vi "lv_icon.vi"(10 "Color icon in":T2, 11 "BW icon in":T2) -> (0 "Error code out":i32=43, 2 "Color icon out":T2, 3 "BW icon out":T2)   [LabVIEW 2020, in "lv_icon.lvlib"]
doc: "<p>Display this dialog box in one of the following ways:</p>\n\n<ul>\n<li>Double-click the <a href=\"nihelplauncher://docs/csh?context=lvcore_lvconcepts_using_icons\">icon</a> in the upper right corner of the front panel window, block diagram window, or <a href=\"nihelplauncher://docs/csh?context=lvcore_lvconcepts_custom_cont_ind_type\">Control Editor</a> window.</li>\n<li>Right-click the icon in the upper right corner of the front panel window, block diagram window, or <strong>Control Editor</strong> window and select <strong>Edit Icon</strong> from the shortcut menu.</li>\n<li>Select <strong>File<span class=\"U+187\">>></span>VI Properties</strong> or <strong>File<span class=\"U+187\">>></span>Control Properties</strong> to display the <a href=\"nihelplauncher://docs/csh?context=lvcore_lvdialog_vi_properties_dialog_box\">VI Properties</a> dialog box or <strong>Control Properties</strong> dialog box, respectively. Then select <strong>General</strong> from the <strong>Category</strong> pull-down menu and click the <strong>Edit Icon</strong> button.</li>\n<li>Right-click a project library, statechart, class, or XControl item in the <a href=\"nihelplauncher://docs/csh?context=lvcore_lvconcepts_using_labview_projects\">Project Explorer</a> window and select <strong> Properties</strong> from the shortcut menu to display the corresponding <strong>Properties</strong> dialog box. Then click the <strong>Edit</strong> button on the <strong>General Settings</strong> page.</li>\n</ul>\n\n<p>Use this dialog box to <a href=\"nihelplauncher://docs/csh?context=lvcore_lvhowto_creating_icons\">create and edit icons</a>.</p>"
uses:
  lv_icon.lvlib
  NIIconEditor/Class/Ants/Ants.lvclass
  NIIconEditor/Class/FakedArray/FakedArray.lvclass
  vi.lib/LabVIEW Icon API/lv_icon/Classes/Icon/Icon.lvclass
  NIIconEditor/Class/Icon Library/Glyph.lvclass
  NIIconEditor/Class/Settings/Settings.lvclass
  NIIconEditor/Class/Tools/Tools Paint.lvclass
  vi.lib/LabVIEW Icon API/lv_icon/Controls/Pathes.ctl
  NIIconEditor/History/History.lvlib
  <vilib>/Utility/miscctls.llb/LVPoint32TypeDef.ctl
  NIIconEditor/Controls/Tools.ctl
  NIIconEditor/Controls/References Cluster.ctl
  NIIconEditor/Controls/Path&Icon.ctl
  vi.lib/LabVIEW Icon API/lv_icon/Controls/Graphic.ctl
  NIIconEditor/Global Variables/Data.vi
  <vilib>/Utility/miscctls.llb/LVMenuShortCut.ctl
  <resource>/plugins/IconEditor/Icon Editor Invoker Type.ctl
  NIIconEditor/Controls/Circle.ctl
  NIIconEditor/Controls/Dropper.ctl
  NIIconEditor/Controls/FCircle.ctl
  NIIconEditor/Controls/Fill.ctl
  NIIconEditor/Controls/FRect.ctl
  NIIconEditor/Controls/Line.ctl
  NIIconEditor/Controls/Move.ctl
  NIIconEditor/Controls/Pen.ctl
  NIIconEditor/Controls/Rubber.ctl
  NIIconEditor/Controls/Selection.ctl
  NIIconEditor/Controls/Text.ctl
  NIIconEditor/Controls/Rotate.ctl
  NIIconEditor/Controls/Flip.ctl
  vi.lib/LabVIEW Icon API/lv_icon/Controls/IEColor.ctl
  NIIconEditor/Controls/ColorChange.ctl
  NIIconEditor/Controls/Framework Templates.ctl
  NIIconEditor/Controls/TextMarker.ctl
  <vilib>/picture/picture.llb/imagedata.ctl
  vi.lib/LabVIEW Icon API/lv_icon/Controls/BodyText.ctl
  vi.lib/LabVIEW Icon API/lv_icon/Controls/Layer.ctl
  vi.lib/LabVIEW Icon API/lv_icon/Controls/Font.ctl
  NIIconEditor/Controls/LayerList.ctl
  vi.lib/LabVIEW Icon API/lv_icon/Controls/Alignment.ctl
  NIIconEditor/Controls/Arrow Up.ctl
  NIIconEditor/Controls/Arrow Down.ctl
  NIIconEditor/Controls/DeleteLayer.ctl
  NIIconEditor/Controls/NewLayer.ctl
  NIIconEditor/Controls/IERect.ctl
  NIIconEditor/Controls/Refresh.ctl
panel:
  out "LabVIEW Icon out":string
  in  "LabVIEW Icon in":string
  out "Terminals":picture
  out "Preview2":picture
  out "TextMarker":T1="^"
  in  "Help":bool
  in  "Cancel":bool
  in  "OK":bool
  out "XYZ":string="X: 14\nY: 31\nZ: 1"
  out "RGB":string="R: 0\nG: 0\nB: 0"
  out "Icon":picture
  out "Clipboard":picture
  in  "Tab Control":T3(tab)
  in  "refreshTemplates":T4
  out "templates path str":string
  in  "Templates":string(tree)="<All>"
  in  "Filter templates by keyword":string
  in  "Framework Templates":T5={"Scrollbar"=0, "Path & Icon 1"={"Rectangle"={"left"=0, "top"=0, "right"=32, "bottom"=32}, "Path"=path "C:/Users/tsandris/Documents/LabVIEW Data/Icon Templates/VI/Frameworks/_blank.png", "Image"=bytes[0], "Filter"="VI\\Frameworks", "FileName"="_blank"}, "Path & Icon 2"={"Rectangle"={"left"=0, "top"=0, "right"=32, "bottom"=32}, "Path"=path "C:/Users/tsandris/Documents/LabVIEW Data/Icon Templates/Library/Frameworks/_blank.png", "Image"=bytes[0], "Filter"="Library\\Frameworks", "FileName"="_blank"}, "Path & Icon 3"={"Rectangle"={"left"=0, "top"=0, "right"=0, "bottom"=0}, "Path"=path "", "Image"=bytes[0], "Filter"="", "FileName"=""}, "Path & Icon 4"={"Rectangle"={"left"=0, "top"=0, "right"=0, "bottom"=0}, "Path"=path "", "Image"=bytes[0], "Filter"="", "FileName"=""}, "Path & Icon 5"={"Rectangle"={"left"=0, "top"=0, "right"=0, "bottom"=0}, "Path"=path "", "Image"=bytes[0], "Filter"="", "FileName"=""}, "Path & Icon 6"={"Rectangle"={"left"=0, "top"=0, "right"=0, "bottom"=0}, "Path"=path "", "Image"=bytes[0], "Filter"="", "FileName"=""}, "Path & Icon 7"={"Rectangle"={"left"=0, "top"=0, "right"=0, "bottom"=0}, "Path"=path "", "Image"=bytes[0], "Filter"="", "FileName"=""}, "Path & Icon 8"={"Rectangle"={"left"=0, "top"=0, "right"=0, "bottom"=0}, "Path"=path "", "Image"=bytes[0], "Filter"="", "FileName"=""}, "Path & Icon 9"={"Rectangle"={"left"=0, "top"=0, "right"=0, "bottom"=0}, "Path"=path "", "Image"=bytes[0], "Filter"="", "FileName"=""}, "Path & Icon 10"={"Rectangle"={"left"=0, "top"=0, "right"=0, "bottom"=0}, "Path"=path "", "Image"=bytes[0], "Filter"="", "FileName"=""}, "Path & Icon 11"={"Rectangle"={"left"=0, "top"=0, "right"=0, "bottom"=0}, "Path"=path "", "Image"=bytes[0], "Filter"="", "FileName"=""}, "Path & Icon 12"={"Rectangle"={"left"=0, "top"=0, "right"=0, "bottom"=0}, "Path"=path "", "Image"=bytes[0], "Filter"="", "FileName"=""}, "Path & Icon 13"={"Rectangle"={"left"=0, "top"=0, "right"=0, "bottom"=0}, "Path"=path "", "Image"=bytes[0], "Filter"="", "FileName"=""}, "Path & Icon 14"={"Rectangle"={"left"=0, "top"=0, "right"=0, "bottom"=0}, "Path"=path "", "Image"=bytes[0], "Filter"="", "FileName"=""}, "Path & Icon 15"={"Rectangle"={"left"=0, "top"=0, "right"=0, "bottom"=0}, "Path"=path "", "Image"=bytes[0], "Filter"="", "FileName"=""}, "Path & Icon 16"={"Rectangle"={"left"=0, "top"=0, "right"=0, "bottom"=0}, "Path"=path "", "Image"=bytes[0], "Filter"="", "FileName"=""}, "Path & Icon 17"={"Rectangle"={"left"=0, "top"=0, "right"=0, "bottom"=0}, "Path"=path "", "Image"=bytes[0], "Filter"="", "FileName"=""}, "Path & Icon 18"={"Rectangle"={"left"=0, "top"=0, "right"=0, "bottom"=0}, "Path"=path "", "Image"=bytes[0], "Filter"="", "FileName"=""}, "Path & Icon 19"={"Rectangle"={"left"=0, "top"=0, "right"=0, "bottom"=0}, "Path"=path "", "Image"=bytes[0], "Filter"="", "FileName"=""}, "Path & Icon 20"={"Rectangle"={"left"=0, "top"=0, "right"=0, "bottom"=0}, "Path"=path "", "Image"=bytes[0], "Filter"="", "FileName"=""}, "Path & Icon 21"={"Rectangle"={"left"=0, "top"=0, "right"=0, "bottom"=0}, "Path"=path "", "Image"=bytes[0], "Filter"="", "FileName"=""}, "Path & Icon 22"={"Rectangle"={"left"=0, "top"=0, "right"=0, "bottom"=0}, "Path"=path "", "Image"=bytes[0], "Filter"="", "FileName"=""}, "Path & Icon 23"={"Rectangle"={"left"=0, "top"=0, "right"=0, "bottom"=0}, "Path"=path "", "Image"=bytes[0], "Filter"="", "FileName"=""}, "Path & Icon 24"={"Rectangle"={"left"=0, "top"=0, "right"=0, "bottom"=0}, "Path"=path "", "Image"=bytes[0], "Filter"="", "FileName"=""}, "Path & Icon 25"={"Rectangle"={"left"=0, "top"=0, "right"=0, "bottom"=0}, "Path"=path "", "Image"=bytes[0], "Filter"="", "FileName"=""}, "Path & Icon 26"={"Rectangle"={"left"=0, "top"=0, "right"=0, "bottom"=0}, "Path"=path "", "Image"=bytes[0], "Filter"="", "FileName"=""}, "Path & Icon 27"={"Rectangle"={"left"=0, "top"=0, "right"=0, "bottom"=0}, "Path"=path "", "Image"=bytes[0], "Filter"="", "FileName"=""}, "Path & Icon 28"={"Rectangle"={"left"=0, "top"=0, "right"=0, "bottom"=0}, "Path"=path "", "Image"=bytes[0], "Filter"="", "FileName"=""}, "Path & Icon 29"={"Rectangle"={"left"=0, "top"=0, "right"=0, "bottom"=0}, "Path"=path "", "Image"=bytes[0], "Filter"="", "FileName"=""}, "Path & Icon 30"={"Rectangle"={"left"=0, "top"=0, "right"=0, "bottom"=0}, "Path"=path "", "Image"=bytes[0], "Filter"="", "FileName"=""}}
  in  "Body Text":T7={"Line 1 text"="", "Line 2 text"="", "Line 3 text"="", "Line 4 text"="", "Line 1 color"=0, "Line 2 color"=0, "Line 3 color"=0, "Line 4 color"=0, "Body Text Spec"={"Font"="", "Alignment"=1, "Size"=9}, "Center text vertically"=TRUE, "Capitalize Text"=TRUE} {"Body Text Spec"."Alignment" items=["left", "center", "right"]}
  in  "Filter glyphs by keyword":string
  in  "Glyphs":string(tree)="<All>"
  out "glyph path str":string
  out "Glyphs []":T6[][](array[typedef])
  in  "refreshGlyphs":T4
  in  "Add Layer":T10
  in  "Remove Layer":T11
  in  "Move Down":T12
  in  "Move Up":T13
  in  "Icon Template":T14={"LayerIcon"=bytes[0], "LayerName"="", "Opacity"=100, "Visibility?"=TRUE} {"Opacity" scale=0.0..100.0}
  in  "Icon Text":T14={"LayerIcon"=bytes[0], "LayerName"="Icon Text", "Opacity"=100, "Visibility?"=TRUE} {"Opacity" scale=0.0..100.0}
  in  "User Layers":T15={"Scrollbar"=0, "Layer 1"={"LayerIcon"=bytes[0], "LayerName"="VI Icon", "Opacity"=100, "Visibility?"=TRUE}, "Layer 2"={"LayerIcon"=bytes[3230], "LayerName"="", "Opacity"=100, "Visibility?"=TRUE}, "Layer 3"={"LayerIcon"=bytes[3230], "LayerName"="", "Opacity"=100, "Visibility?"=TRUE}, "Layer 4"={"LayerIcon"=bytes[3230], "LayerName"="", "Opacity"=100, "Visibility?"=TRUE}} {"Layer 4"."Opacity" scale=0.0..100.0; "Layer 3"."Opacity" scale=0.0..100.0; "Layer 2"."Opacity" scale=0.0..100.0; "Layer 1"."Opacity" scale=0.0..100.0}
  out "Preview":picture
  in  "Horizontal Flip":T16
  in  "Clockwise Rotate":T17
  in  "Swap":T18
  in  "Line Color":T19
  in  "Fill Color":T19=16777215
  in  "Tools":T20=enum."Rectangle"
  # "Clipboard control. Anything made on this\ncontrol will show up in the clipboard image data."
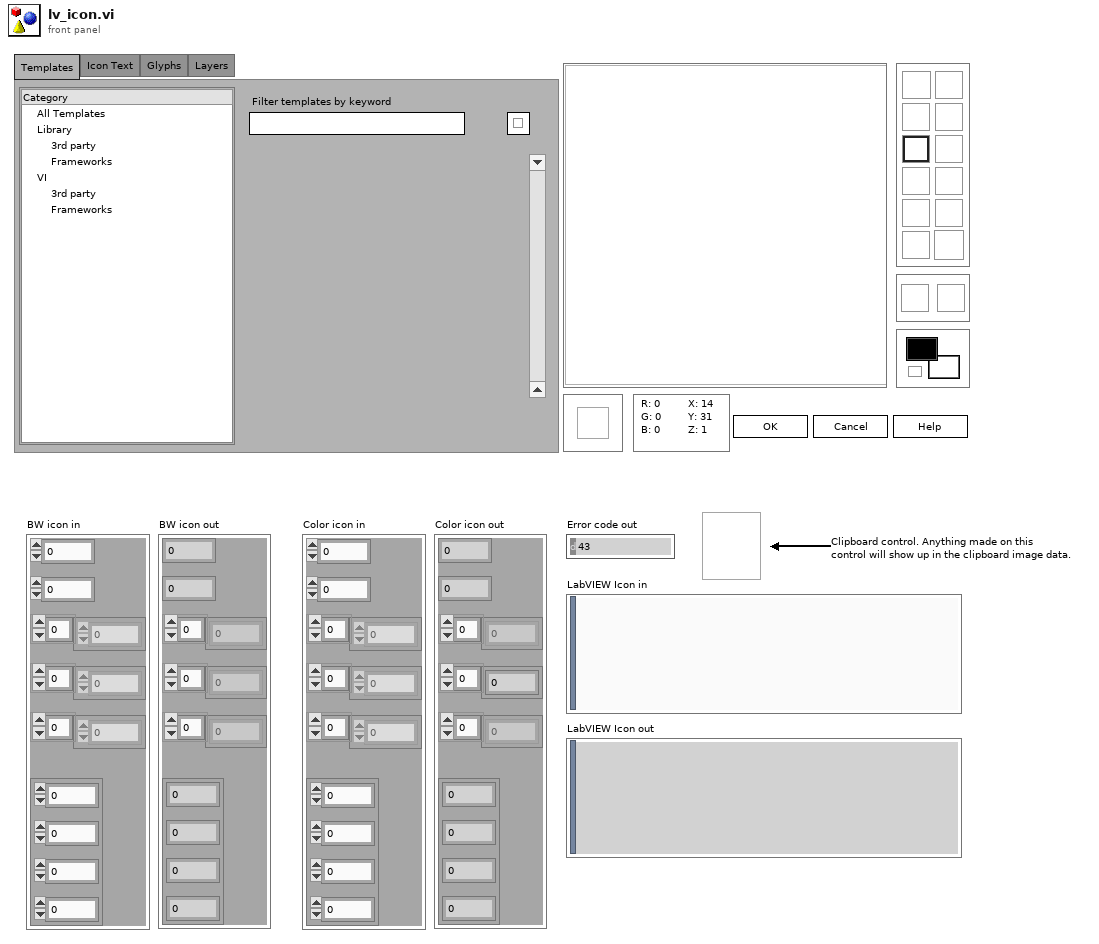
[diagram p1: front panel]
types:
  T1 = typedef "TextMarker.ctl" = string
  T2 = typedef "imagedata.ctl" = cluster{"image type":i32, "image depth":i32, "image":u8[], "mask":u8[], "colors":u32[], "Rectangle":cluster{"left":i16, "top":i16, "right":i16, "bottom":i16}}
  T3 = enum32{"Templates", "Icon Text", "Glyphs", "Layers"}
  T4 = typedef "Refresh.ctl" = bool
  T5 = typedef "Framework Templates.ctl" = cluster{"Scrollbar":i32, "Path & Icon 1":T6, "Path & Icon 2":T6, "Path & Icon 3":T6, "Path & Icon 4":T6, "Path & Icon 5":T6, "Path & Icon 6":T6, "Path & Icon 7":T6, "Path & Icon 8":T6, "Path & Icon 9":T6, "Path & Icon 10":T6, "Path & Icon 11":T6, "Path & Icon 12":T6, "Path & Icon 13":T6, "Path & Icon 14":T6, "Path & Icon 15":T6, "Path & Icon 16":T6, "Path & Icon 17":T6, "Path & Icon 18":T6, "Path & Icon 19":T6, "Path & Icon 20":T6, "Path & Icon 21":T6, "Path & Icon 22":T6, "Path & Icon 23":T6, "Path & Icon 24":T6, "Path & Icon 25":T6, "Path & Icon 26":T6, "Path & Icon 27":T6, "Path & Icon 28":T6, "Path & Icon 29":T6, "Path & Icon 30":T6}
  T6 = typedef "Graphic.ctl" = cluster{"Rectangle":cluster{"left":i16, "top":i16, "right":i16, "bottom":i16}, "Path":path, "Image":picture, "Filter":string, "FileName":string}
  T7 = typedef "BodyText.ctl" = cluster{"Line 1 text":string, "Line 2 text":string, "Line 3 text":string, "Line 4 text":string, "Line 1 color":u32, "Line 2 color":u32, "Line 3 color":u32, "Line 4 color":u32, "Body Text Spec":cluster{"Font":T8, "Alignment":T9, "Size":u8}, "Center text vertically":bool, "Capitalize Text":bool}
  T8 = typedef "Font.ctl" = string
  T9 = typedef "Alignment.ctl" = u16
  T10 = typedef "NewLayer.ctl" = bool
  T11 = typedef "DeleteLayer.ctl" = bool
  T12 = typedef "Arrow Down.ctl" = bool
  T13 = typedef "Arrow Up.ctl" = bool
  T14 = typedef "Layer.ctl" = cluster{"LayerIcon":picture, "LayerName":string, "Opacity":u8, "Visibility?":bool}
  T15 = typedef "LayerList.ctl" = cluster{"Scrollbar":i32, "Layer 1":T14, "Layer 2":T14, "Layer 3":T14, "Layer 4":T14}
  T16 = typedef "Flip.ctl" = bool
  T17 = typedef "Rotate.ctl" = bool
  T18 = typedef "ColorChange.ctl" = bool
  T19 = typedef "IEColor.ctl" = u32
  T20 = typedef "Tools.ctl" = enum32{"Pencil", "Line", "Dropper", "Fill", "Rectangle", "Filled Rectangle", "Ellipse", "Filled Ellipse", "Eraser", "Text", "Select", "Move"}
  T21 = typedef "Icon Editor Invoker Type.ctl" = enum32{"Unknown Icon Source", "VI Icon", "Library Icon (any library type)", "Palette icon", "Icon from App Method"}
  T22 = enum32{"Invalid", "Default", "Floating", "Floating/Auto-Hide", "Modal"}
  T23 = enum32{"Invalid", "Standard", "Closed", "Hidden", "Minimized", "Maximized"}
  T24 = typedef "lv_icon.lvlib/References Cluster.ctl" = cluster{"Add Layer":refnum<vi>, "Remove Layer":refnum<vi>, "Line Text":refnum<vi>[], "Body Text Spec":refnum<vi>, "DNL_Font":refnum<vi>, "glyph path str":refnum<vi>, "templates path str":refnum<vi>, "Arrow Up":refnum<vi>, "Arrow Down":refnum<vi>, "IE VI Ref":refnum<vi>, "Glyphs tree":refnum<vi>, "Templates tree":refnum<vi>, "Layer Icon Text":refnum<vi>, "Layer Template":refnum<vi>, "Body Text":refnum<vi>, "Search Templates":refnum<vi>, "TextMarker":refnum<vi>, "Tab Control":refnum<vi>, "Search Glyphs":refnum<vi>, "Line Color":refnum<vi>, "DNL_Glyphs []":refnum<vi>, "Fill Color":refnum<vi>, "Tools":refnum<vi>, "Icon":refnum<vi>, "Preview":refnum<vi>, "Ants":refnum<vi>, "Terminals":refnum<vi>, "menu reference":refnum<k9>, "LayerNames":refnum<vi>[], "GlyphLoadAnimation":refnum<vi>, "TemplateLoadAnimation":refnum<vi>, "refreshGlyphs":refnum<vi>, "refreshTemplates":refnum<vi>}
  T25 = typedef "Who Invoked Icon Editor.ctl" = cluster{"Icon Editor Invoker Type":T21, "App Refnum of Invoker":refnum<vi>, "Qualified Name of Invoker":string, "Path to Invoker":path}
  T26 = typedef "LVMenuShortCut.ctl" = cluster{"Include Shift Key?":bool, "Include Ctrl Key?":bool, "Shortcut Key":string}
  T27 = cluster{"Global stop?":refnum<user-event>, "Templates":refnum<user-event>, "Glyphs":refnum<user-event>}
  T28 = typedef "lv_icon.lvlib/Global Data.ctl" = cluster{"Class":T29, "Ref":T24, "Support":T30}
  T29 = typedef "lv_icon.lvlib/IE Classes.ctl" = cluster{"Ants":refnum<class "Ants.lvclass">, "Layer":refnum<class "FakedArray.lvclass">, "Templates":refnum<class "FakedArray.lvclass">, "Icon":refnum<class "Icon.lvclass">, "Glyph":refnum<class "Glyph.lvclass">, "Settings":refnum<class "Settings.lvclass">, "Tools":refnum<class "Tools Paint.lvclass">, "History":refnum<class "History.lvclass">}
  T30 = typedef "lv_icon.lvlib/Support Cluster.ctl" = cluster{"AntsRect":cluster{"left":i16, "top":i16, "right":i16, "bottom":i16}, "Mouse Move Coords":T31, "Mouse Down Coords":T31, "Temp Coord":T31, "Action":T32, "Edge Color":T19, "Fill Color":T19, "Mouse Down?":bool, "Draft Mode?":bool, "Temp Icon":picture, "CTRL Pressed":bool, "Move Selection?":bool, "AntsRect Orig":cluster{"left":i16, "top":i16, "right":i16, "bottom":i16}, "Text":string, "TM Set?":bool, "Mouse inside icon?":bool, "Tool (old value)":u32, "Pencil Move Color":u32, "Swap Colors?":bool, "Shift pressed?":bool}
  T31 = typedef "LVPoint32TypeDef.ctl" = cluster{"Horizontal":i32, "Vertical":i32}
  T32 = typedef "SupportClass_Action.ctl" = enum16{"Default", "Move Selection", "Glyph Library", "Tool"}
  T33 = typedef "Pathes.ctl" = enum16{"Root Path", "Icon Templates", "Icon Templates VI", "Icon Templates Lib", "Glyphs"}
  T34 = typedef "Path&Icon.ctl" = cluster{"Rectangle":cluster{"left":i16, "top":i16, "right":i16, "bottom":i16}, "Path":path, "Image":picture, "Filter":string, "FileName":string}
  T35 = typedef "lveventtype.ctl" = enum32{"Null", "Timeout", "Annotation Menu Selection", "Annotation Menu Selection?", "App Instance Close", "App Instance Close?", "Autoscale Range Change", "Bookmark Info Change", "Cell Edit", "Cell Edit?", "Cursor Grab", "Cursor Grab?", "Cursor Menu Selection", "Cursor Menu Selection?", "Cursor Move", "Cursor Release", "Data Change", "Direction Change", "Display State Change", "Drag Ended", "Drag Enter", "Drag Leave", "Drag Over", "Drag Source Update", "Drag Starting", "Drag Starting?", "Drop", "Exec State Change", "Key Down", "Key Down?", "Key Repeat", "Key Repeat?", "Key Up", "Listbox Double Click", "Menu Activation?", "Menu Selection (App)", "Menu Selection? (App)", "Menu Selection (User)", "Mouse Down", "Mouse Down?", "Mouse Enter", "Mouse Leave", "Mouse Move", "Mouse Up", "Mouse Wheel", "NI Security User Change (App)", "Pane Size", "Panel Close", "Panel Close?", "Panel Resize", "Plot Attribute Change", "Scale Range Change", "Shortcut Menu Activation?", "Shortcut Menu Selection (App)", "Shortcut Menu Selection? (App)", "Shortcut Menu Selection (User)", "Tree Double Click", "Tree Drag", "Tree Drag?", "Tree Drop", "Tree Drop?", "Tree Item Close", "Tree Item Close?", "Tree Item Open", "Tree Item Open?", "URL Change?", "User Event", "Value Change"}
  T36 = typedef "eventvkey.ctl" = enum16{"ASCII", "Enter", "Return", "Shift", "Ctrl", "Alt", "Cmd", "Opt", "Caps", "NumLock", "Clear", "Break", "Up", "Down", "Left", "Right", "Insert", "Delete", "Home", "End", "PageUp", "PageDown", "Escape", "Help", "Pause", "ScrollLock", "F1", "F2", "F3", "F4", "F5", "F6", "F7", "F8", "F9", "F10", "F11", "F12", "F13", "F14", "F15", "F16", "F17", "F18", "F19", "F20", "F21", "F22", "F23", "F24", "Play", "VolumeUp", "VolumeDown", "Mute", "Two Byte Char"}
  T37 = cluster{"Shift":bool, "Ctrl":bool, "Alt":bool, "Cmd":bool, "Opt":bool}
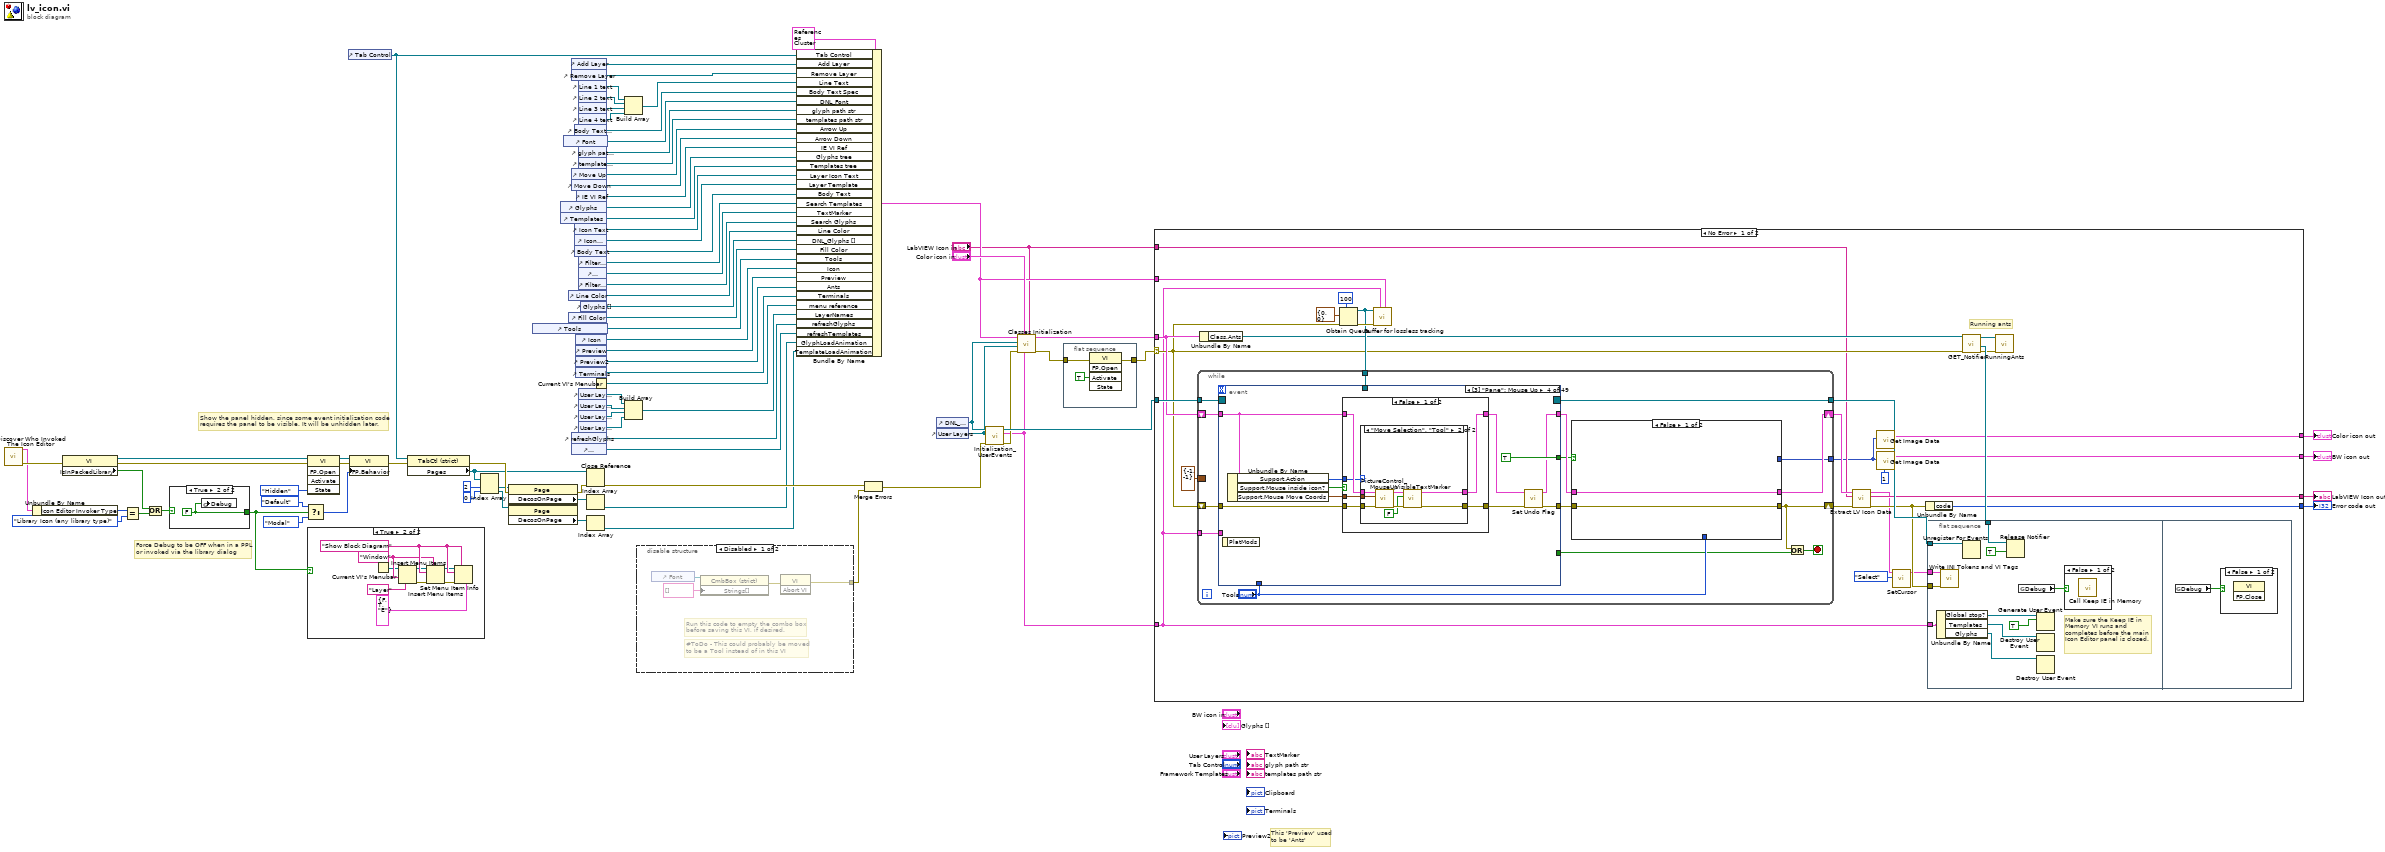
[diagram p0: block diagram]
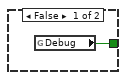
[diagram p2: hidden frame]
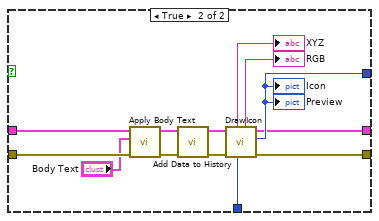
[diagram p5: hidden frame]
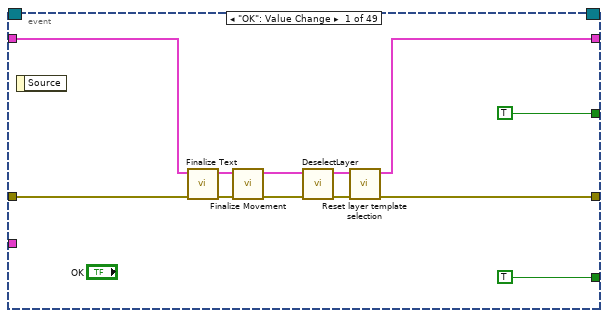
[diagram p6: hidden frame]
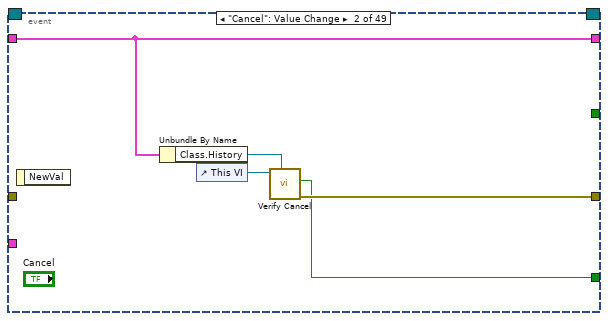
[diagram p7: hidden frame]
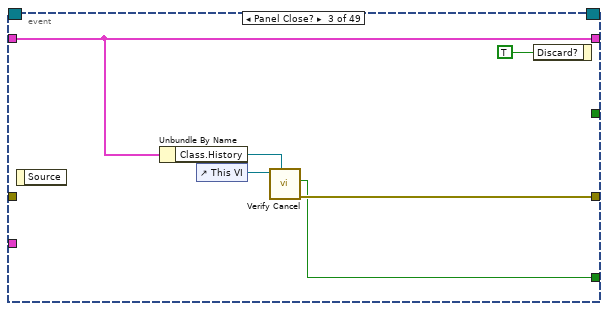
[diagram p8: hidden frame]
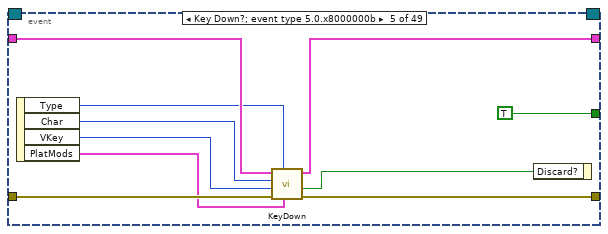
[diagram p11: hidden frame]
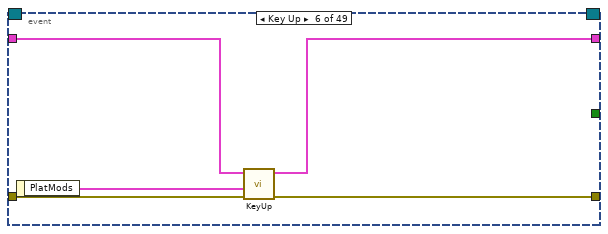
[diagram p12: hidden frame]
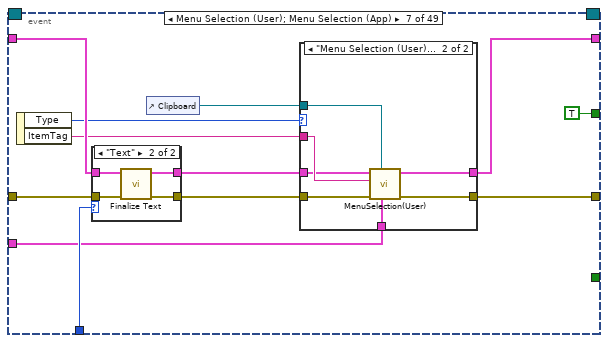
[diagram p13: hidden frame]
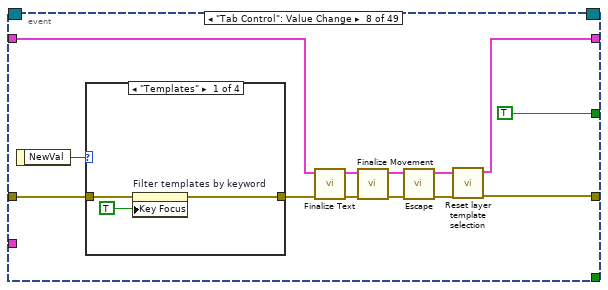
[diagram p16: hidden frame]
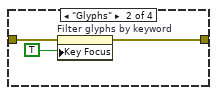
[diagram p17: hidden frame]
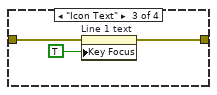
[diagram p18: hidden frame]
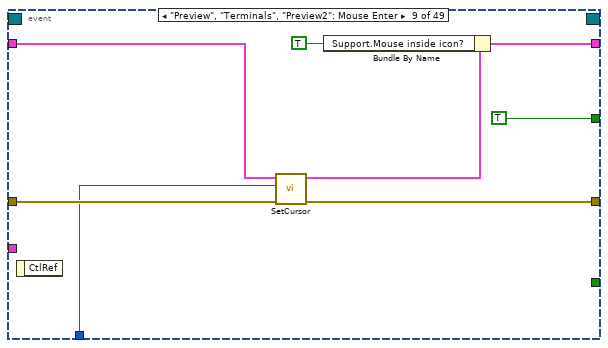
[diagram p20: hidden frame]
diagram:
  # "Force Debug to be OFF when in a PPL\nor invoked via the library dialog"
  # "Show the panel hidden, since some event initialization code requires the panel to be visible. It will be unhidden later."
  # "This 'Preview' used\nto be 'Ants'"
  n1 = call <resource>:"Discover Who Invoked The Icon Editor.vi"() -> ("error out"=w7:errorcluster, "Who Invoked The Icon Editor?"=w6:T25)  [unwired: 10 in]
  n2 = Unbundle By Name(w6) -> ("Icon Editor Invoker Type"=w5:T21)
  n3 = property class="VI"(error in=w7) -> (reference out=w9:refnum<vi>, error out=w8:errorcluster, "IsInPackedLibrary"=w2:bool)  [unwired: 1 in]
  n4 = Equal?(x=w5, y=Icon_Editor_Invoker_Type."Library Icon (any library type)") -> (x = y?=w3:bool)
  n5 = Or(x=w2, y=w3) -> (x .or. y?=w1:bool)
  n6 = case shown="True" w1 {
    tunnel: [w87 w88] -> w10
    frame False {
      n7 = global read "Data.vi" "Debug"() -> (w87:bool)
    }
    frame True {
      w88 = FALSE
      n8 = global write "Data.vi" "Debug"(w88) -> ()
    }
  }
  n9 = Select(t=T22."Default" ("Front Panel Window:Behavior"), s=w10, f=T22."Modal" ("Front Panel Window:Behavior")) -> (s? t:f=w11:T22)
  n10 = invoke class="VI" method="FP.Open"(reference=w9, error in=w8, "State"=T23."Hidden") -> (reference out=w14:refnum<vi>, error out=w16:errorcluster)  [unwired: 2 in, 3 out]
  n11 = case shown="True" w10 {
    frame False {
    }
    frame True {
      w97 = "Show Block Diagram"
      w92 = "Window" ("menu tag")
      n12 = Current VI's Menubar() -> (w89:refnum<k9>)
      n13 = Insert Menu Items(4:"Layer" ("after item"), 7:w92, 9:w89) -> (0:w94:errorcluster, 3:w95:refnum<k9>)  [unwired: 3 in, 1 out]
      n14 = Insert Menu Items(5:w92, 6:w94, 8:w97, 9:w95) -> (0:w90:errorcluster, 3:w91:refnum<k9>)  [unwired: 2 in, 1 out]
      n15 = Set Menu Item Info(4:T26 {"Include Shift Key?"=FALSE, "Include Ctrl Key?"=TRUE, "Shortcut Key"="E"} ("short cut"), 7:w97, 8:w90, 10:w97, 11:w91) -> ()  [unwired: 2 in, 2 out]
    }
  }
  n16 = control-ref of="Tab Control"() -> (w19:refnum<vi>)
  n17 = property class="VI"(reference=w14, error in=w16, "FP.Behavior"=w11) -> (error out=w15:errorcluster)  [unwired: 1 out]
  n18 = property class="TabCtl (strict)"(reference=w19, error in=w15) -> (error out=w29:errorcluster, "Pages"=w21:refnum<vi>[])  [unwired: 1 out]
  n19 = Index Array(array=w21, index #1=2 ("index"), index #2=0 ("index")) -> (element #1=w25:refnum<vi>, element #2=w26:refnum<vi>)
  n20 = property class="Page"(reference=w25, error in=w29) -> (error out=w22:errorcluster, "DecosOnPage"=w24:refnum<vi>[])  [unwired: 1 out]
  n21 = property class="Page"(reference=w26) -> ("DecosOnPage"=w23:refnum<vi>[])  [unwired: 1 in, 2 out]
  n22 = control-ref of="Tools"() -> (w83:refnum<vi>)
  n23 = control-ref of="Glyphs"() -> (w67:refnum<vi>)
  n24 = control-ref of="Templates"() -> (w68:refnum<vi>)
  n25 = control-ref of="Font"() -> (w49:refnum<vi>)
  n26 = control-ref of="Line Color"() -> (w81:refnum<vi>)
  n27 = control-ref of="Fill Color"() -> (w82:refnum<vi>)
  n28 = control-ref of="Add Layer"() -> (w52:refnum<vi>)
  n29 = control-ref of="Remove Layer"() -> (w53:refnum<vi>)
  n30 = control-ref of="Move Up"() -> (w64:refnum<vi>)
  n31 = control-ref of="Move Down"() -> (w65:refnum<vi>)
  n32 = control-ref of="refreshGlyphs"() -> (w39:refnum<vi>)
  n33 = control-ref of="refreshTemplates"() -> (w40:refnum<vi>)
  n34 = control-ref of="Body Text Spec"() -> (w61:refnum<vi>)
  n35 = control-ref of="Icon Text"() -> (w70:refnum<vi>)
  n36 = control-ref of="Icon Template"() -> (w71:refnum<vi>)
  n37 = control-ref of="Body Text"() -> (w76:refnum<vi>)
  n38 = control-ref of="Icon"() -> (w84:refnum<vi>)
  n39 = control-ref of="Preview"() -> (w85:refnum<vi>)
  n40 = control-ref of="Preview2"() -> (w60:refnum<vi>)
  n41 = control-ref of="Terminals"() -> (w75:refnum<vi>)
  n42 = control-ref of="IE VI Ref"() -> (w66:refnum<vi>)
  n43 = control-ref of="Line 1 text"() -> (w55:refnum<vi>)
  n44 = control-ref of="Line 2 text"() -> (w56:refnum<vi>)
  n45 = control-ref of="Line 3 text"() -> (w57:refnum<vi>)
  n46 = control-ref of="Line 4 text"() -> (w58:refnum<vi>)
  n47 = control-ref of="glyph path str"() -> (w62:refnum<vi>)
  n48 = control-ref of="templates path str"() -> (w63:refnum<vi>)
  n49 = control-ref of="Filter templates by keyword"() -> (w78:refnum<vi>)
  n50 = control-ref of="TextMarker"() -> (w79:refnum<vi>)
  n51 = control-ref of="Filter glyphs by keyword"() -> (w80:refnum<vi>)
  n52 = control-ref of="User Layer 1"() -> (w44:refnum<vi>)
  n53 = control-ref of="User Layer 2"() -> (w45:refnum<vi>)
  n54 = control-ref of="User Layer 3"() -> (w46:refnum<vi>)
  n55 = control-ref of="User Layer 4"() -> (w47:refnum<vi>)
  n56 = control-ref of="Glyphs []"() -> (w50:refnum<vi>)
  n57 = Close Reference(reference=w21, error in (no error)=w22) -> (error out=w20:errorcluster)
  n58 = Index Array(array=w24) -> (element=w18:refnum<vi>)  [unwired: 1 in]
  n59 = Index Array(array=w23) -> (element=w17:refnum<vi>)  [unwired: 1 in]
  n60 = Current VI's Menubar() -> (w74:refnum<k9>)
  n61 = Build Array(w55, w56, w57, w58) -> (w54:refnum<vi>[])
  n62 = Build Array(w44, w45, w46, w47) -> (w42:refnum<vi>[])
  n63 = disable-structure shown="Disabled" {
    disable-tunnel: [w98 _] -> w31
    frame Disabled {
      # "#ToDo - This could probably be moved\nto be a Tool instead of in this VI"
      # "Run this code to empty the combo box\nbefore saving this VI, if desired."
      n64 = control-ref of="Font"() -> (w101:refnum<vi>)
      n65 = property class="CmbBox (strict)"(reference=w101, "Strings[]"=string[] [] ("Strings []")) -> (error out=w99:errorcluster)  [unwired: 1 in, 1 out]
      n66 = invoke class="VI" method="Abort VI"(error in=w99) -> (error out=w98:errorcluster)  [unwired: 2 in, 2 out]
    }
    frame Enabled {
    }
  }
  n67 = Bundle By Name(cluster=T24 {"Add Layer"=refnum, "Remove Layer"=refnum, "Line Text"=[], "Body Text Spec"=refnum, "DNL_Font"=refnum, "glyph path str"=refnum, "templates path str"=refnum, "Arrow Up"=refnum, "Arrow Down"=refnum, "IE VI Ref"=refnum, "Glyphs tree"=refnum, "Templates tree"=refnum, "Layer Icon Text"=refnum, "Layer Template"=refnum, "Body Text"=refnum, "Search Templates"=refnum, "TextMarker"=refnum, "Tab Control"=refnum, "Search Glyphs"=refnum, "Line Color"=refnum, "DNL_Glyphs []"=refnum, "Fill Color"=refnum, "Tools"=refnum, "Icon"=refnum, "Preview"=refnum, "Ants"=refnum, "Terminals"=refnum, "menu reference"=refnum, "LayerNames"=[], "GlyphLoadAnimation"=refnum, "TemplateLoadAnimation"=refnum, "refreshGlyphs"=refnum, "refreshTemplates"=refnum} ("references"), "Tab Control"=w19, "Add Layer"=w52, "Remove Layer"=w53, "Line Text"=w54, "Body Text Spec"=w61, "DNL_Font"=w49, "glyph path str"=w62, "templates path str"=w63, "Arrow Up"=w64, "Arrow Down"=w65, "IE VI Ref"=w66, "Glyphs tree"=w67, "Templates tree"=w68, "Layer Icon Text"=w70, "Layer Template"=w71, "Body Text"=w76, "Search Templates"=w78, "TextMarker"=w79, "Search Glyphs"=w80, "Line Color"=w81, "DNL_Glyphs []"=w50, "Fill Color"=w82, "Tools"=w83, "Icon"=w84, "Preview"=w85, "Ants"=w60, "Terminals"=w75, "menu reference"=w74, "LayerNames"=w42, "refreshGlyphs"=w39, "refreshTemplates"=w40, "GlyphLoadAnimation"=w18, "TemplateLoadAnimation"=w17) -> (w43:T24)
  n68 = Merge Errors(w20, w31) -> (w30:errorcluster)
  n69 = control-ref of="DNL_Framework Templates"() -> (w33:refnum<vi>)
  n70 = control-ref of="User Layers"() -> (w32:refnum<vi>)
  n71 = call "Initialization_UserEvents.vi"("error in"=w30, "Layer Clusters"=w32, "DNL_Framework Templates"=w33) -> ("error out"=w72:errorcluster, "User events"=w34:T27, "Events"=w77:refnum<event-registration>)  [unwired: 6 out]
  n72 = call "Classes Initialization.vi"("LabVIEW Icon in"="LabVIEW Icon in", "User events"=w34, "Color icon in"="Color icon in", "error in"=w72, "Layer Clusters"=w32, "DNL_Framework Templates"=w33, "Ref Cluster"=w43) -> ("error out"=w36:errorcluster, "Data out"=w59:T28)  [unwired: 3 out]
  n73 = flat-sequence {
    tunnel: w36 -> [w103]
    tunnel: [w102] -> w35
    frame #0 {
      n74 = invoke class="VI" method="FP.Open"(error in=w103, "Activate"=TRUE ("Activate?")) -> (error out=w102:errorcluster)  [unwired: 3 in, 4 out]
    }
  }
  n75 = case shown="No Error" w35 {
    selector: w35 -> [w115 w803]
    tunnel: w77 -> [w131 _]
    tunnel: [w129 w804] -> w73
    tunnel: [w127 _] -> w69
    tunnel: w34 -> [w106 _]
    tunnel: w59 -> [w120 _]
    tunnel: w43 -> [w118 _]
    tunnel: [w117 _] -> w51
    tunnel: "LabVIEW Icon in" -> [w110 w802]
    tunnel: [w113 w802] -> w48
    frame No Error {
      # "Running ants"
      n76 = Unbundle By Name(w120) -> ("Class.Ants"=w119:refnum<class "Ants.lvclass">)
      n77 = Obtain Queue(max queue size (-1, unlimited)=100, element data type=T31 {"Horizontal"=0, "Vertical"=0} ("Coords"), error in (no error)=w115) -> (queue out=w121:refnum<queue>, error out=w122:errorcluster)  [unwired: 1 in, 2 out]
      n78 = while {
        shift-right: [w133] -> w112
        shift-left: w115 -> [w144]
        tunnel: [w141] -> w132
        tunnel: w131 -> [w140]
        tunnel: [w139] -> w105
        tunnel: w121 -> [w136]
        shift-right: [w146] -> w114
        shift-left: w120 -> [w135]
        border: T31 {"Horizontal"=-1, "Vertical"=-1} ("Corrected Out") -> [_]
        tunnel: w106 -> [w134]
        stop <- w142 stop-if-true
        n79 = event shown="[3] \"Pane\": Mouse Up" {
          selector: w140 -> [_ _ _ _ _ _ _ _ _ _ _ _ _ _ _ _ _ _ _ _ _ _ _ _ _ _ _ _ _ _ _ _ _ _ _ _ _ _ _ _ _ _ _ _ _ _ _ _ _]
          dyn-events: [_ _ _ _ _ _ _ _ _ _ _ _ _ _ _ _ _ _ _ _ _ _ _ _ _ _ _ _ _ _ _ _ _ _ _ _ _ _ _ _ _ _ _ _ _ _ _ _ _] -> w141
          timeout: _ -> [_ _ _ _ _ _ _ _ _ _ _ _ _ _ _ _ _ _ _ _ _ _ _ _ _ _ _ _ _ _ _ _ _ _ _ _ _ _ _ _ _ _ _ _ _ _ _ _ _]
          tunnel: [w168 w179 w185 w188 w222 w228 w231 w264 w285 w295 w308 w325 w329 w335 w339 w348 w360 w374 w389 w400 w425 w432 w444 w461 w482 w491 w508 w528 w533 w537 w544 w549 w572 w588 w603 w614 w627 w646 w660 w682 w695 w710 w720 w722 w741 w758 w778 w785 w787] -> w138
          tunnel: w144 -> [w170 _ _ w193 w223 w227 w237 w266 w286 w296 w308 w326 w332 w337 w342 w352 w359 w368 w391 w409 w426 w435 w448 w463 w485 w504 w516 w529 w534 w538 w545 w563 w576 w591 w607 w615 w633 w649 w662 w685 w703 w713 w719 w731 w748 w762 w779 w785 w788]
          tunnel: [TRUE w178 w184 _ _ _ _ _ _ _ _ _ _ _ _ _ _ _ _ _ _ _ _ _ _ _ _ _ _ _ _ _ _ _ _ _ _ _ _ _ _ _ _ _ _ _ _ _ _] -> w143
          tunnel: "Tools" -> [_ _ _ _ _ _ w235 _ w284 _ _ _ _ _ _ _ _ _ _ _ _ _ _ _ _ _ _ _ _ _ _ _ _ _ _ _ _ _ _ _ _ _ _ _ _ _ _ _ _]
          tunnel: [TRUE _ _ TRUE ("Yes") TRUE _ TRUE TRUE TRUE TRUE _ TRUE TRUE _ TRUE TRUE TRUE TRUE TRUE TRUE _ _ TRUE TRUE _ TRUE ("Yes") _ _ _ _ TRUE TRUE TRUE _ TRUE _ TRUE TRUE ("Yes") TRUE TRUE _ _ _ _ TRUE ("Yes") TRUE _ _ _] -> w137
          tunnel: w136 -> [_ _ _ _ _ _ _ _ _ w293 _ _ _ _ _ _ _ _ _ _ _ _ _ _ _ _ _ _ _ _ _ _ _ _ _ _ _ _ _ _ _ _ _ _ _ _ _ _ _]
          tunnel: w135 -> [w167 w176 w182 w192 w218 w226 w240 w262 w282 w292 w305 w322 w328 w334 w341 w351 w358 w370 w384 w396 w429 w431 w441 w459 w478 w495 w513 w526 w536 w540 w542 w548 w569 w586 w599 w612 w625 w651 w669 w680 w693 w709 w717 w727 w746 w755 w776 w784 w789]
          tunnel: [w163 w176 w182 w186 w215 w224 w232 w256 w280 w291 w307 w321 w327 w333 w344 w346 w356 w373 w385 w401 w414 w430 w439 w457 w477 w489 w509 w526 w536 w539 w541 w547 w567 w585 w598 w611 w624 w639 w653 w679 w697 w708 w715 w723 w740 w752 w776 w784 w789] -> w147
          tunnel: w134 -> [_ _ _ _ _ _ w230 _ _ _ _ _ _ _ _ _ _ _ _ _ _ _ _ _ _ _ _ w527 _ _ _ _ _ _ _ _ _ _ _ _ _ _ _ _ _ _ w777 _ _]
          event "OK": Value Change {
            n80 = event-data() -> ()  [unwired: 2 out]
            n81 = call "Finalize Text.vi"("error in (no error)"=w170, "Data in"=w167) -> ("error out"=w171:errorcluster, "Data out"=w166:T28)  [unwired: 8 out]
            n82 = call "Finalize Movement.vi"("error in (no error)"=w171, "Data in"=w166) -> ("error out"=w172:errorcluster, "Data out"=w165:T28)  [unwired: 1 in, 7 out]
            n83 = call "DeselectLayer.vi"("error in (no error)"=w172, "Data in"=w165) -> ("error out"=w169:errorcluster, "Data out"=w164:T28)  [unwired: 8 out]
            n84 = call "Reset layer template selection.vi"("error in (no error)"=w169, "Data in"=w164) -> ("error out"=w168:errorcluster, "Data out"=w163:T28)  [unwired: 1 in, 7 out]
          }
          event "Cancel": Value Change {
            n85 = event-data() -> ()  [unwired: 2 out]
            n86 = Unbundle By Name(w176) -> ("Class.History"=w175:refnum<class "History.lvclass">)
            n87 = control-ref of="This VI"() -> (w177:refnum<vi>)
            n88 = call "Verify Cancel.vi"("History"=w175, "Calling VI"=w177) -> ("error out"=w179:errorcluster, "Close IE"=w178:bool)  [unwired: 8 in]
          }
          event Panel Close? {
            n89 = event-data() -> ()  [unwired: 2 out]
            n90 = Unbundle By Name(w182) -> ("Class.History"=w181:refnum<class "History.lvclass">)
            n91 = control-ref of="This VI"() -> (w183:refnum<vi>)
            n92 = call "Verify Cancel.vi"("History"=w181, "Calling VI"=w183) -> ("error out"=w185:errorcluster, "Close IE"=w184:bool)  [unwired: 8 in]
            n93 = event-data("Discard?"=TRUE) -> ()  [unwired: 1 in, 1 out]
          }
          event Mouse Up {
            n94 = event-data() -> ()  [unwired: 2 out]
            n95 = Unbundle By Name(w192) -> ("Support.Action"=w190:T32, "Support.Mouse inside icon?"=w195:bool, "Support.Mouse Move Coords"=w191:T31)
            n96 = case shown="False" w195 {
              tunnel: w193 -> [w199 w213]
              tunnel: [w197 w213] -> w189
              tunnel: [w200 w212] -> w187
              tunnel: w192 -> [w201 w212]
              tunnel: w191 -> [w198 _]
              tunnel: w190 -> [w196 _]
              frame False {
                n97 = case shown="\"Move Selection\", \"Tool\"" w196 {
                  tunnel: w201 -> [w203 w210]
                  tunnel: [w203 w205] -> w200
                  tunnel: w199 -> [w202 w209]
                  tunnel: w198 -> [_ w211]
                  tunnel: [w202 w206] -> w197
                  frame "Default", Default {
                  }
                  frame "Move Selection", "Tool" {
                    n98 = call "PictureControl_MouseUp.vi"("error in"=w209, "Coords"=w211, "Data in"=w210) -> ("error out"=w207:errorcluster, "Data out"=w208:T28)  [unwired: 4 in, 3 out]
                    n99 = call "VisibleTextMarker.vi"("error in"=w207, "Visible"=FALSE, "Data in"=w208) -> ("error out"=w206:errorcluster, "Data out"=w205:T28)  [unwired: 7 in]
                  }
                }
              }
              frame True {
              }
            }
            n100 = call "Set Undo Flag.vi"("error in"=w189, "Data in"=w187) -> ("error out"=w188:errorcluster, "Data out"=w186:T28)  [unwired: 8 in]
          }
          event Key Down?; event type 5.0.x8000000b {
            n101 = event-data() -> ("Type"=w217:T35, "Char"=w214:i16, "VKey"=w221:T36, "PlatMods"=w216:T37)  [unwired: 1 out]
            n102 = call "KeyDown.vi"("PlatMods"=w216, "Type"=w217, "error in (no error)"=w223, "VKey"=w221, "Char"=w214, "Data in"=w218) -> ("error out"=w222:errorcluster, "Discard?"=w220:bool, "Data out"=w215:T28)  [unwired: 3 out]
            n103 = event-data("Discard?"=w220) -> ()  [unwired: 1 in, 1 out]
          }
          event Key Up {
            n104 = event-data() -> ("PlatMods"=w225:T37)  [unwired: 1 out]
            n105 = call "KeyUp.vi"("error in (no error)"=w227, "PlatMods"=w225, "Data in"=w226) -> ("error out"=w228:errorcluster, "Data out"=w224:T28)  [unwired: 7 out]
          }
          event Menu Selection (User); Menu Selection (App) {
            n106 = event-data() -> ("Type"=w238:T35, "ItemTag"=w239:string)  [unwired: 1 out]
            n107 = case shown="\"Text\"" w235 {
              tunnel: w237 -> [w241 w246]
              tunnel: w240 -> [w242 w245]
              tunnel: [w241 w244] -> w233
              tunnel: [w242 w243] -> w234
              frame Default {
              }
              frame "Text" {
                n108 = call "Finalize Text.vi"("error in (no error)"=w246, "Data in"=w245) -> ("error out"=w244:errorcluster, "Data out"=w243:T28)  [unwired: 8 out]
              }
            }
            n109 = control-ref of="Clipboard"() -> (w229:refnum<vi>)
            n110 = case shown="\"Menu Selection (User)\"" w238 {
              tunnel: w239 -> [_ w255]
              tunnel: [w248 w254] -> w231
              tunnel: w233 -> [w248 w253]
              tunnel: w230 -> [_ w252]
              tunnel: w234 -> [w247 w251]
              tunnel: [w247 w250] -> w232
              tunnel: w229 -> [_ w249]
              frame Default {
              }
              frame "Menu Selection (User)" {
                n111 = call "MenuSelection(User).vi"("User events"=w252, "Clipboard"=w249, "error in"=w253, "ItemTag"=w255, "Data in"=w251) -> ("error out"=w254:errorcluster, "Data out"=w250:T28)  [unwired: 5 out]
              }
            }
          }
          event "Tab Control": Value Change {
            n112 = event-data() -> ("NewVal"=w267:T3)  [unwired: 1 out]
            n113 = case shown="\"Templates\"" w267 {
              tunnel: w266 -> [w271 w274 w276 w278]
              tunnel: [w270 w273 w277 w278] -> w265
              frame "Templates" {
                n114 = property on="Filter templates by keyword" class="Str"(error in=w271, "Key Focus"=TRUE) -> (error out=w270:errorcluster)  [unwired: 1 in, 1 out]
              }
              frame "Glyphs" {
                n115 = property on="Filter glyphs by keyword" class="Str"(error in=w274, "Key Focus"=TRUE) -> (error out=w273:errorcluster)  [unwired: 1 in, 1 out]
              }
              frame "Icon Text" {
                n116 = property on="Line 1 text" class="Str"(error in=w276, "Key Focus"=TRUE) -> (error out=w277:errorcluster)  [unwired: 1 in, 1 out]
              }
              frame "Layers", Default {
              }
            }
            n117 = call "Finalize Text.vi"("error in (no error)"=w265, "Data in"=w262) -> ("error out"=w268:errorcluster, "Data out"=w261:T28)  [unwired: 8 out]
            n118 = call "Finalize Movement.vi"("error in (no error)"=w268, "Data in"=w261) -> ("error out"=w260:errorcluster, "Data out"=w258:T28)  [unwired: 1 in, 7 out]
            n119 = call "Escape.vi"("error in"=w260, "Data in"=w258) -> ("error out"=w259:errorcluster, "Data out"=w257:T28)  [unwired: 1 in, 7 out]
            n120 = call "Reset layer template selection.vi"("error in (no error)"=w259, "Data in"=w257) -> ("error out"=w264:errorcluster, "Data out"=w256:T28)  [unwired: 1 in, 7 out]
          }
          event "Preview", "Terminals", "Preview2": Mouse Enter {
            n121 = event-data() -> ()  [unwired: 2 out]
            n122 = call "SetCursor.vi"("error in (no error)"=w286, "Radio Buttons"=w284, "Data in"=w282) -> ("error out"=w285:errorcluster, "Data out"=w281:T28)  [unwired: 7 out]
            n123 = Bundle By Name(cluster=w281, "Support.Mouse inside icon?"=TRUE) -> (w280:T28)
          }
          event "Preview", "Terminals", "Preview2": Mouse Move {
            n124 = event-data() -> ("Coords"=w290:T31)  [unwired: 1 out]
            n125 = call "CoordinatesCorrection.vi"("Coordinates In"=w290) -> ("Corrected Out"=w287:T31)  [unwired: 10 out]
            n126 = feedback-in #1(w287) -> ()
            n127 = feedback #1() -> (w289:T31)
            n128 = Not Equal?(x=w289, y=w287) -> (x != y?=w288:bool)
            n129 = case shown="True" w288 {
              tunnel: w296 -> [w298 w304]
              tunnel: [w298 w303] -> w295
              tunnel: w293 -> [_ w302]
              tunnel: w292 -> [w297 w301]
              tunnel: [w297 w300] -> w291
              tunnel: w287 -> [_ w299]
              frame False {
              }
              frame True {
                n130 = call "MouseMove.vi"("Buffer"=w302, "error in"=w304, "Coords"=w299, "Data in"=w301) -> ("error out"=w303:errorcluster, "Data out"=w300:T28)  [unwired: 6 out]
              }
            }
          }
          event "Preview", "Preview2", "Terminals": Mouse Leave {
            n131 = event-data() -> ()  [unwired: 2 out]
            n132 = Bundle By Name(cluster=w305, "Support.Mouse inside icon?"=FALSE) -> (w307:T28)
          }
          event "Preview", "Terminals", "Preview2": Mouse Down {
            # "Left click"
            n133 = event-data() -> ("Button"=w311:u16, "Coords"=w324:T31)  [unwired: 1 out]
            n134 = Not Equal?(x=u16 1, y=w311) -> (x != y?=w309:bool)
            n135 = control-ref of="This VI"() -> (w320:refnum<vi>)
            n136 = call "Defer_FP_Updates.vi"("Defer Panel Updates"=TRUE, "error in"=w326, "lv_icon.vi in"=w320) -> ("error out"=w316:errorcluster, "lv icon.vi out"=w318:refnum<vi>)  [unwired: 7 out]
            n137 = call "Reset layer template selection.vi"("Force reset? (T)"=FALSE, "error in (no error)"=w316, "Data in"=w322) -> ("error out"=w315:errorcluster, "Data out"=w312:T28)  [unwired: 1 in, 6 out]
            n138 = call "MouseDown.vi"("Flip colors?"=w309, "error in"=w315, "Coords"=w324, "Data in"=w312) -> ("error out"=w314:errorcluster, "Data out"=w321:T28)  [unwired: 1 in, 5 out]
            n139 = call "Defer_FP_Updates.vi"("Defer Panel Updates"=FALSE, "error in"=w314, "lv_icon.vi in"=w318) -> ("error out"=w325:errorcluster)  [unwired: 8 out]
          }
          event "Preview", "Terminals", "Preview2": Mouse Up {
            n140 = event-data() -> ("Coords"=w331:T31)  [unwired: 1 out]
            n141 = call "PictureControl_MouseUp.vi"("error in"=w332, "Coords"=w331, "Data in"=w328) -> ("error out"=w329:errorcluster, "Data out"=w327:T28)  [unwired: 4 in, 3 out]
          }
          event Value Change {
            n142 = event-data() -> ("NewVal"=w336:T20)  [unwired: 1 out]
            n143 = call "Value Change_Tools.vi"("error in"=w337, "NewVal"=w336, "Data in"=w334) -> ("error out"=w335:errorcluster, "Data out"=w333:T28)  [unwired: 7 out]
          }
          event Mouse Down {
            n144 = event-data() -> ("Mods.Double Click"=w338:bool)  [unwired: 1 out]
            n145 = call "Mouse Down.vi"("error in"=w342, "Double Click"=w338, "Data in"=w341) -> ("error out"=w339:errorcluster, "Data out"=w340:T28)  [unwired: 7 out]
            n146 = Bundle By Name(cluster=w340, "Support.Tool (old value)"=u32 111) -> (w344:T28)
          }
          event Mouse Down {
            n147 = event-data() -> ()  [unwired: 2 out]
            n148 = call "Finalize Text.vi"("error in (no error)"=w352, "Data in"=w351) -> ("error out"=w353:errorcluster, "Data out"=w350:T28)  [unwired: 8 out]
            n149 = call "Finalize Movement.vi"("error in (no error)"=w353, "Data in"=w350) -> ("error out"=w349:errorcluster, "Data out"=w347:T28)  [unwired: 1 in, 7 out]
            n150 = call "Escape.vi"("error in"=w349, "Data in"=w347) -> ("error out"=w348:errorcluster, "Data out"=w346:T28)  [unwired: 1 in, 7 out]
          }
          event Value Change {
            n151 = event-data() -> ()  [unwired: 2 out]
            n152 = call "Check Color.vi"("Color in"="Fill Color") -> ("Color out"=w361:T19)  [unwired: 26 out]
            n153 = call "Check Color.vi"("Color in"="Line Color") -> ("Color out"=w362:T19)  [unwired: 26 out]
            n154 = Bundle By Name(cluster=w358, "Support.Fill Color"=w361, "Support.Edge Color"=w362) -> (w357:T28)
            n155 = call "Escape.vi"("Reset cursor (T)"=FALSE ("Reset cursor? (T)"), "error in"=w359, "Data in"=w357) -> ("error out"=w360:errorcluster, "Data out"=w356:T28)  [unwired: 1 in, 6 out]
          }
          event Value Change {
            n156 = event-data() -> ()  [unwired: 2 out]
            n157 = call "Finalize Text.vi"("error in (no error)"=w368, "Data in"=w370) -> ("error out"=w372:errorcluster, "Data out"=w371:T28)  [unwired: 8 out]
            n158 = local read "Line Color"() -> (w367:T19)
            n159 = local read "Fill Color"() -> (w377:T19)
            n160 = call "Finalize Movement.vi"("error in (no error)"=w372, "Data in"=w371) -> ("error out"=w366:errorcluster, "Data out"=w369:T28)  [unwired: 1 in, 7 out]
            n161 = stacked-sequence {
              tunnel: w377 -> [w381]
              tunnel: [w380] -> w375
              tunnel: w367 -> [w379]
              tunnel: w366 -> [w378]
              frame #0 {
                n162 = local write "Fill Color"(w379) -> ()
                n163 = property on="Line Color" class="ColBox (strict)"(error in=w378, "Val(Sgnl)"=w381) -> (error out=w380:errorcluster)  [unwired: 1 in, 1 out]
              }
            }
            n164 = call "Escape.vi"("error in"=w375, "Data in"=w369) -> ("error out"=w374:errorcluster, "Data out"=w373:T28)  [unwired: 1 in, 7 out]
          }
          event Value Change {
            n165 = event-data() -> ()  [unwired: 2 out]
            n166 = call "Finalize Text.vi"("error in (no error)"=w391, "Data in"=w384) -> ("error out"=w390:errorcluster, "Data out"=w386:T28)  [unwired: 8 out]
            n167 = call "Finalize Movement.vi"("error in (no error)"=w390, "Data in"=w386) -> ("error out"=w387:errorcluster, "Data out"=w383:T28)  [unwired: 1 in, 7 out]
            n168 = call "RotateFlip.vi"("error in"=w387, "Rotate"="Clockwise Rotate", "Data in"=w383) -> ("error out"=w388:errorcluster, "Data out"=w382:T28)  [unwired: 2 in, 5 out]
            n169 = call "Escape.vi"("error in"=w388, "Data in"=w382) -> ("error out"=w389:errorcluster, "Data out"=w385:T28)  [unwired: 1 in, 7 out]
          }
          event User Event {
            # "This is an initialization event for the templates"
            n170 = event-data() -> ("Templates"=w411:string)  [unwired: 1 out]
            n171 = Unbundle By Name(w396) -> ("Ref.TemplateLoadAnimation"=w395:refnum<vi>, "Ref.refreshTemplates"=w394:refnum<vi>)
            n172 = control-ref of="This VI"() -> (w406:refnum<vi>)
            n173 = call "Defer_FP_Updates.vi"("Defer Panel Updates"=TRUE, "error in"=w409, "lv_icon.vi in"=w406) -> ("error out"=w404:errorcluster, "lv icon.vi out"=w403:refnum<vi>)  [unwired: 7 out]
            n174 = Unflatten From String(type=cluster{T6[], i32, bool} {[], 0, FALSE}, binary string=w411, error in (no error)=w404) -> (value=w402:cluster{T6[], i32, bool}, error out=w407:errorcluster)  [unwired: 3 out]
            n175 = call "Process Template Graphics.vi"("error in (no error)"=w407, "Data"=w402, "Data in"=w396) -> ("error out"=w399:errorcluster, "Data out"=w401:T28)  [unwired: 7 out]
            n176 = call "ChangeRefreshGraphicsState.vi"("error in (no error)"=w399, "refreshing?"=FALSE, "button ref"=w394, "animatedDecoration ref"=w395) -> ("error out"=w398:errorcluster)  [unwired: 7 in]
            n177 = call "Defer_FP_Updates.vi"("error in"=w398, "lv_icon.vi in"=w403) -> ("error out"=w400:errorcluster)  [unwired: 1 in, 8 out]
          }
          event "Templates": Value Change {
            # "Templates Category Tree"
            n178 = event-data() -> ("CtlRef"=w413:refnum<vi>, "NewVal"=w424:string)  [unwired: 1 out]
            n179 = control-ref of="This VI"() -> (w428:refnum<vi>)
            n180 = Unbundle By Name(w429) -> ("Class.Templates"=w416:refnum<class "FakedArray.lvclass">)
            n181 = call "Defer_FP_Updates.vi"("Defer Panel Updates"=TRUE, "error in"=w426, "lv_icon.vi in"=w428) -> ("error out"=w418:errorcluster, "lv icon.vi out"=w423:refnum<vi>)  [unwired: 7 out]
            n182 = call-dynamic "SET_ScrollbarPosition.vi"("error in (no error)"=w418, "FakedArray.lvclass in"=w416) -> ("error out"=w420:errorcluster, "FakedArray.lvclass out"=w419:refnum<class "FakedArray.lvclass">)  [unwired: 1 in, 7 out]
            n183 = local write "Filter templates by keyword"("") -> ()
            n184 = call "ResetColor.vi"("error in (no error)"=w420, "FakedArray in"=w419) -> ("error out"=w421:errorcluster, "FakedArray out"=w422:refnum<class "FakedArray.lvclass">)  [unwired: 8 out]
            n185 = call-dynamic "UpdateVisibleData.vi"("Templates tree"=w413, "error in (no error)"=w421, "Tag"=w424, "FakedArray in"=w422) -> ("error out"=w417:errorcluster, "FakedArray out"=w415:refnum<class "FakedArray.lvclass">)  [unwired: 1 in, 5 out]
            n186 = Bundle By Name(cluster=w429, "Class.Templates"=w415) -> (w414:T28)
            n187 = call "Defer_FP_Updates.vi"("error in"=w417, "lv_icon.vi in"=w423) -> ("error out"=w425:errorcluster)  [unwired: 1 in, 8 out]
          }
          event "Templates": Mouse Down {
            n188 = event-data() -> ("CtlRef"=w434:refnum<vi>, "Coords"=w436:T31)  [unwired: 1 out]
            n189 = call "Mouse Down_Tree.vi"("Tree"=w434, "error in (no error)"=w435, "Coords"=w436) -> ("error out"=w433:errorcluster)  [unwired: 8 out]
            n190 = call "Escape.vi"("error in"=w433, "Data in"=w431) -> ("error out"=w432:errorcluster, "Data out"=w430:T28)  [unwired: 1 in, 7 out]
          }
          event Value Change {
            n191 = event-data() -> ("OldVal.Opacity"=w442:u8, "NewVal.Opacity"=w443:u8)  [unwired: 1 out]
            n192 = Equal?(x=w442, y=w443) -> (x = y?=w437:bool)
            n193 = call "Value Change_Top or Bottom Layer.vi"("Type"=enum16{"Template Layer", "Text Layer"}."Template Layer", "error in (no error)"=w448, "Data"="Icon Template", "Data in"=w441) -> ("error out"=w445:errorcluster, "Data out"=w440:T28)  [unwired: 6 out]
            n194 = case shown="False" w437 {
              tunnel: w445 -> [w450 w453]
              tunnel: [w449 w456] -> w444
              tunnel: w440 -> [w452 w454]
              tunnel: [w451 w455] -> w439
              frame False {
                # "Opacity changed"
                n195 = call "Reset layer template selection.vi"("error in (no error)"=w450, "Data in"=w452) -> ("error out"=w449:errorcluster, "Data out"=w451:T28)  [unwired: 1 in, 7 out]
              }
              frame True {
                # "Opacity did not change"
                n196 = call "Set Undo Flag.vi"("error in"=w453, "Data in"=w454) -> ("error out"=w456:errorcluster, "Data out"=w455:T28)  [unwired: 8 in]
              }
            }
          }
          event Mouse Down {
            n197 = event-data() -> ("CtlRef"=w462:refnum<vi>, "Button"=w458:u16)  [unwired: 1 out]
            n198 = case shown="1, 2" w458 {
              tunnel: w463 -> [w465 w471]
              tunnel: w462 -> [_ w475]
              tunnel: [w465 w470] -> w461
              tunnel: w459 -> [w464 w468]
              tunnel: [w464 w467] -> w457
              frame 0, Default {
              }
              frame 1, 2 {
                n199 = control-ref of="This VI"() -> (w474:refnum<vi>)
                n200 = call "Defer_FP_Updates.vi"("Defer Panel Updates"=TRUE, "error in"=w471, "lv_icon.vi in"=w474) -> ("error out"=w472:errorcluster, "lv icon.vi out"=w469:refnum<vi>)  [unwired: 7 out]
                n201 = call "Template_MouseDown.vi"("Add to Undo?"=TRUE, "error in"=w472, "CtlRef"=w475, "Data in"=w468) -> ("error out"=w476:errorcluster, "Data out"=w467:T28)  [unwired: 1 in, 5 out]
                n202 = call "Defer_FP_Updates.vi"("error in"=w476, "lv_icon.vi in"=w469) -> ("error out"=w470:errorcluster)  [unwired: 1 in, 8 out]
              }
            }
          }
          event Value Change {
            n203 = event-data() -> ("NewVal"=w487:variant)  [unwired: 1 out]
            n204 = control-ref of="This VI"() -> (w484:refnum<vi>)
            n205 = call "Defer_FP_Updates.vi"("Defer Panel Updates"=TRUE, "error in"=w485, "lv_icon.vi in"=w484) -> ("error out"=w486:errorcluster, "lv icon.vi out"=w479:refnum<vi>)  [unwired: 7 out]
            n206 = call "Mouse Down_Templates.vi"("Tag"="Templates", "error in"=w486, "NewVal"=w487, "Data in"=w478) -> ("error out"=w481:errorcluster, "Data out"=w477:T28)  [unwired: 1 in, 5 out]
            n207 = call "Defer_FP_Updates.vi"("error in"=w481, "lv_icon.vi in"=w479) -> ("error out"=w482:errorcluster)  [unwired: 1 in, 8 out]
          }
          event "Filter templates by keyword": Value Change {
            n208 = event-data() -> ("NewVal"=w507:string)  [unwired: 1 out]
            n209 = Unbundle By Name(w495) -> ("Ref.Templates tree"=w493:refnum<vi>, "Class.Templates"=w496:refnum<class "FakedArray.lvclass">)
            n210 = control-ref of="This VI"() -> (w506:refnum<vi>)
            n211 = call "Defer_FP_Updates.vi"("Defer Panel Updates"=TRUE, "error in"=w504, "lv_icon.vi in"=w506) -> ("error out"=w498:errorcluster, "lv icon.vi out"=w503:refnum<vi>)  [unwired: 7 out]
            n212 = call-dynamic "SET_ScrollbarPosition.vi"("error in (no error)"=w498, "FakedArray.lvclass in"=w496) -> ("error out"=w499:errorcluster, "FakedArray.lvclass out"=w500:refnum<class "FakedArray.lvclass">)  [unwired: 1 in, 7 out]
            n213 = call "ResetColor.vi"("error in (no error)"=w499, "FakedArray in"=w500) -> ("error out"=w501:errorcluster, "FakedArray out"=w502:refnum<class "FakedArray.lvclass">)  [unwired: 8 out]
            n214 = call-dynamic "UpdateVisibleData.vi"("Templates tree"=w493, "error in (no error)"=w501, "Keyword"=w507, "FakedArray in"=w502) -> ("error out"=w497:errorcluster, "FakedArray out"=w494:refnum<class "FakedArray.lvclass">)  [unwired: 1 in, 5 out]
            n215 = Bundle By Name(cluster=w495, "Class.Templates"=w494) -> (w490:T28)
            n216 = call "Defer_FP_Updates.vi"("error in"=w497, "lv_icon.vi in"=w503) -> ("error out"=w492:errorcluster)  [unwired: 1 in, 8 out]
            n217 = call "Set Undo Flag.vi"("error in"=w492, "Data in"=w490) -> ("error out"=w491:errorcluster, "Data out"=w489:T28)  [unwired: 8 in]
          }
          event "Filter templates by keyword": Mouse Down {
            # "If a mouse down event should\nselect the entered text, enable this case"
            n218 = event-data() -> ("CtlRef"=w517:refnum<vi>)  [unwired: 1 out]
            n219 = disable-structure shown="Disabled" {
              disable-tunnel: w517 -> [w522 _]
              disable-tunnel: w516 -> [w520 w523]
              disable-tunnel: [w518 w523] -> w515
              frame Disabled {
                n220 = property class="Str"(reference=w522, error in=w520, "Text.Selection Start"=u32 0 ("Text.Selection:Start"), "Text.Selection End"=-1 ("Text.Selection:End")) -> (error out=w518:errorcluster)  [unwired: 1 out]
              }
              frame Enabled {
              }
            }
            n221 = call "Finalize Text.vi"("error in (no error)"=w515, "Data in"=w513) -> ("error out"=w514:errorcluster, "Data out"=w512:T28)  [unwired: 8 out]
            n222 = call "DeselectLayer.vi"("error in (no error)"=w514, "Data in"=w512) -> ("error out"=w511:errorcluster, "Data out"=w510:T28)  [unwired: 8 out]
            n223 = call "Escape.vi"("error in"=w511, "Data in"=w510) -> ("error out"=w508:errorcluster, "Data out"=w509:T28)  [unwired: 1 in, 7 out]
          }
          event Value Change {
            n224 = event-data() -> ()  [unwired: 2 out]
            n225 = Unbundle By Name(w526) -> ("Ref.TemplateLoadAnimation"=w524:refnum<vi>, "Ref.refreshTemplates"=w525:refnum<vi>)
            n226 = call "Launch Dynamically Load Graphics.vi"("User events"=w527, "Path"=Pathes."Icon Templates", "error in (no error)"=w529, "button ref"=w525, "animatedDecoration ref"=w524) -> ("error out"=w528:errorcluster)  [unwired: 1 in, 5 out]
          }
          event Mouse Down {
            n227 = event-data() -> ("CtlRef"=w535:refnum<vi>)  [unwired: 1 out]
            n228 = property class="CmbBox (strict)"(reference=w535, error in=w534, "Text.Selection Start"=u32 0 ("Text.Selection:Start"), "Text.Selection End"=u32 1000 ("Text.Selection:End")) -> (error out=w533:errorcluster)  [unwired: 1 out]
          }
          event Mouse Down {
            n229 = event-data() -> ()  [unwired: 2 out]
            n230 = call "Escape.vi"("error in"=w538, "Data in"=w540) -> ("error out"=w537:errorcluster, "Data out"=w539:T28)  [unwired: 1 in, 7 out]
          }
          event Mouse Down {
            n231 = event-data() -> ()  [unwired: 2 out]
            n232 = call "MouseDown_Body Text.vi"("error in"=w545, "Data in"=w542) -> ("error out"=w544:errorcluster, "Data out"=w541:T28)  [unwired: 8 out]
          }
          event Value Change {
            n233 = event-data() -> ("OldVal.Body Text Spec.Font"=w561:T8, "NewVal.Body Text Spec.Font"=w560:T8, "NewVal.Body Text Spec.Alignment"=w555:T9, "OldVal.Body Text Spec.Alignment"=w551:T9)  [unwired: 1 out]
            n234 = local read "Tab Control"() -> (w558:T3)
            n235 = Equal?(x=w558, y=T3."Icon Text") -> (x = y?=w556:bool)
            n236 = Not Equal?(x=w561, y=w560) -> (x != y?=w559:bool)
            n237 = Not Equal?(x=w555, y=w551) -> (x != y?=w553:bool)
            n238 = Or(x=w559, y=w553) -> (x .or. y?=w554:bool)
            n239 = And(x=w556, y=w554) -> (x .and. y?=w546:bool)
            n240 = Unbundle By Name(w548) -> ("Ref.Line Text"=w552:refnum<vi>[])
            n241 = case shown="True" w546 {
              selector: w546 -> [_ w564]
              frame False {
              }
              frame True {
                n242 = property on="Line 1 text" class="Str"("Key Focus"=w564) -> ()  [unwired: 2 in, 2 out]
              }
            }
            n243 = call "Alignment Value Change.vi"("error in"=w563, "NewVal"=w555, "Line Text"=w552) -> ("error out"=w550:errorcluster)  [unwired: 2 in, 6 out]
            n244 = call "Set Undo Flag.vi"("error in"=w550, "Data in"=w548) -> ("error out"=w549:errorcluster, "Data out"=w547:T28)  [unwired: 8 in]
          }
          event Value Change {
            n245 = event-data() -> ("OldVal.Opacity"=w571:u8, "NewVal.Opacity"=w570:u8)  [unwired: 1 out]
            n246 = Equal?(x=w571, y=w570) -> (x = y?=w565:bool)
            n247 = call "Value Change_Top or Bottom Layer.vi"("Type"=enum16{"Template Layer", "Text Layer"}."Text Layer", "error in (no error)"=w576, "Data"="Icon Text", "Data in"=w569) -> ("error out"=w573:errorcluster, "Data out"=w568:T28)  [unwired: 6 out]
            n248 = case shown="False" w565 {
              tunnel: w573 -> [w578 w581]
              tunnel: [w577 w584] -> w572
              tunnel: w568 -> [w580 w582]
              tunnel: [w579 w583] -> w567
              frame False {
                # "Opacity changed"
                n249 = call "Reset layer template selection.vi"("error in (no error)"=w578, "Data in"=w580) -> ("error out"=w577:errorcluster, "Data out"=w579:T28)  [unwired: 1 in, 7 out]
              }
              frame True {
                # "Opacity did not change"
                n250 = call "Set Undo Flag.vi"("error in"=w581, "Data in"=w582) -> ("error out"=w584:errorcluster, "Data out"=w583:T28)  [unwired: 8 in]
              }
            }
          }
          event Value Change {
            n251 = event-data() -> ("NewVal"=w595:variant)  [unwired: 1 out]
            n252 = control-ref of="This VI"() -> (w592:refnum<vi>)
            n253 = call "Defer_FP_Updates.vi"("Defer Panel Updates"=TRUE, "error in"=w591, "lv_icon.vi in"=w592) -> ("error out"=w590:errorcluster, "lv icon.vi out"=w587:refnum<vi>)  [unwired: 7 out]
            n254 = Variant To Data(error in=w590, type=0, Variant=w595) -> (data=w594:i32, error out=w596:errorcluster)
            n255 = call "UpdateLayerView_ScrollbarChanged.vi"("error in"=w596, "Scrollbar Position"=w594, "Data in"=w586) -> ("error out"=w589:errorcluster, "Data out"=w585:T28)  [unwired: 7 out]
            n256 = call "Defer_FP_Updates.vi"("error in"=w589, "lv_icon.vi in"=w587) -> ("error out"=w588:errorcluster)  [unwired: 1 in, 8 out]
          }
          event Mouse Down {
            n257 = event-data() -> ("PlatMods.Shift"=w600:bool, "CtlRef"=w610:refnum<vi>, "PlatMods.Ctrl"=w609:bool)  [unwired: 1 out]
            n258 = control-ref of="This VI"() -> (w606:refnum<vi>)
            n259 = call "Defer_FP_Updates.vi"("Defer Panel Updates"=TRUE, "error in"=w607, "lv_icon.vi in"=w606) -> ("error out"=w605:errorcluster, "lv icon.vi out"=w602:refnum<vi>)  [unwired: 7 out]
            n260 = call "Mouse Down_User Layers.vi"("Shift"=w600, "error in"=w605, "Ctrl"=w609, "CtlRef"=w610, "Data in"=w599) -> ("error out"=w604:errorcluster, "Data out"=w598:T28)  [unwired: 5 out]
            n261 = call "Defer_FP_Updates.vi"("error in"=w604, "lv_icon.vi in"=w602) -> ("error out"=w603:errorcluster)  [unwired: 1 in, 8 out]
          }
          event Mouse Down {
            n262 = event-data() -> ("Button"=w613:u16)  [unwired: 1 out]
            n263 = case shown="1" w613 {
              tunnel: w615 -> [w617 w621]
              tunnel: [w617 w620] -> w614
              tunnel: w612 -> [w616 w619]
              tunnel: [w616 w618] -> w611
              frame 0, Default {
              }
              frame 1 {
                # "Left click"
                n264 = call "Reset layer template selection.vi"("error in (no error)"=w621, "Data in"=w619) -> ("error out"=w620:errorcluster, "Data out"=w618:T28)  [unwired: 1 in, 7 out]
              }
            }
          }
          event Value Change {
            # "We do not use the dynamic registerd event for Layer Clust.Value Change\nbecause it would be a huge effort to lock the front panel until this\nevent case has been completed."
            n265 = event-data() -> ("OldVal.Visibility?"=w623:bool, "CtlRef"=w637:refnum<vi>, "OldVal.LayerName"=w622:string)  [unwired: 1 out]
            n266 = control-ref of="This VI"() -> (w634:refnum<vi>)
            n267 = call "Defer_FP_Updates.vi"("Defer Panel Updates"=TRUE, "error in"=w633, "lv_icon.vi in"=w634) -> ("error out"=w632:errorcluster, "lv icon.vi out"=w629:refnum<vi>)  [unwired: 7 out]
            n268 = call "LayerCluster_ValueChange.vi"("Old Visibility?"=w623, "error in"=w632, "Old name"=w622, "CtlRef"=w637, "Data in"=w625) -> ("error out"=w631:errorcluster, "Data out"=w626:T28)  [unwired: 1 in, 4 out]
            n269 = call "Defer_FP_Updates.vi"("Defer Panel Updates"=FALSE, "error in"=w631, "lv_icon.vi in"=w629) -> ("error out"=w628:errorcluster)  [unwired: 8 out]
            n270 = call "Reset layer template selection.vi"("error in (no error)"=w628, "Data in"=w626) -> ("error out"=w627:errorcluster, "Data out"=w624:T28)  [unwired: 1 in, 7 out]
          }
          event Value Change {
            n271 = event-data() -> ()  [unwired: 2 out]
            n272 = control-ref of="This VI"() -> (w650:refnum<vi>)
            n273 = call "Defer_FP_Updates.vi"("Defer Panel Updates"=TRUE, "error in"=w649, "lv_icon.vi in"=w650) -> ("error out"=w647:errorcluster, "lv icon.vi out"=w640:refnum<vi>)  [unwired: 7 out]
            n274 = call "Add new Layer.vi"("error in"=w647, "Data in"=w651) -> ("error out"=w644:errorcluster, "Data out"=w645:T28)  [unwired: 8 out]
            n275 = call "ViewLayer.vi"("error in (no error)"=w644, "Data in"=w645) -> ("error out"=w643:errorcluster, "Data out"=w641:T28)  [unwired: 2 in, 6 out]
            n276 = call "Set Undo Flag.vi"("error in"=w643, "Data in"=w641) -> ("error out"=w642:errorcluster, "Data out"=w639:T28)  [unwired: 8 in]
            n277 = call "Defer_FP_Updates.vi"("error in"=w642, "lv_icon.vi in"=w640) -> ("error out"=w646:errorcluster)  [unwired: 1 in, 8 out]
          }
          event Value Change {
            n278 = event-data() -> ()  [unwired: 2 out]
            n279 = control-ref of="This VI"() -> (w663:refnum<vi>)
            n280 = Unbundle By Name(w669) -> ("Class.Icon"=w668:refnum<class "Icon.lvclass">)
            n281 = call "Defer_FP_Updates.vi"("Defer Panel Updates"=TRUE, "error in"=w662, "lv_icon.vi in"=w663) -> ("error out"=w661:errorcluster, "lv icon.vi out"=w652:refnum<vi>)  [unwired: 7 out]
            n282 = call-dynamic "GET_All User Layers.vi"("error in (no error)"=w661, "Icon.lvclass in"=w668) -> ("error out"=w675:errorcluster, "User Layer"=w671:refnum<class "Layer.lvclass">[], "Icon.lvclass out"=w670:refnum<class "Icon.lvclass">)  [unwired: 7 out]
            n283 = call "Delete Selected Layers.vi"("error in"=w675, "All Layers in"=w671, "Data in"=w669) -> ("error out"=w674:errorcluster, "All Layers out"=w672:refnum<class "Layer.lvclass">[], "Data out"=w666:T28)  [unwired: 6 in]
            n284 = call-dynamic "SET_UserLayers.vi"("error in"=w674, "Layers"=w672, "Icon.lvclass in"=w670) -> ("error out"=w673:errorcluster, "Icon.lvclass out"=w667:refnum<class "Icon.lvclass">)  [unwired: 7 in]
            n285 = Bundle By Name(cluster=w666, "Class.Icon"=w667) -> (w665:T28)
            n286 = call "Reset layer template selection.vi"("error in (no error)"=w673, "Data in"=w665) -> ("error out"=w657:errorcluster, "Data out"=w658:T28)  [unwired: 1 in, 7 out]
            n287 = call "ViewLayer.vi"("error in (no error)"=w657, "Data in"=w658) -> ("error out"=w656:errorcluster, "Data out"=w654:T28)  [unwired: 3 in, 5 out]
            n288 = call "Set Undo Flag.vi"("error in"=w656, "Data in"=w654) -> ("error out"=w655:errorcluster, "Data out"=w653:T28)  [unwired: 8 in]
            n289 = call "Defer_FP_Updates.vi"("error in"=w655, "lv_icon.vi in"=w652) -> ("error out"=w660:errorcluster)  [unwired: 1 in, 8 out]
          }
          event Value Change {
            n290 = event-data() -> ()  [unwired: 2 out]
            n291 = control-ref of="This VI"() -> (w686:refnum<vi>)
            n292 = call "Defer_FP_Updates.vi"("Defer Panel Updates"=TRUE, "error in"=w685, "lv_icon.vi in"=w686) -> ("error out"=w684:errorcluster, "lv icon.vi out"=w683:refnum<vi>)  [unwired: 7 out]
            n293 = call "MoveLayers.vi"("error in"=w684, "Arrow Up"="Move Up", "Data in"=w680) -> ("error out"=w676:errorcluster, "Data out"=w679:T28)  [unwired: 7 out]
            n294 = stacked-sequence {
              tunnel: [w689] -> w677
              tunnel: w676 -> [w689]
              frame #0 {
                w690 = FALSE ("Arrow Down")
                n295 = local write "Move Down"(w690) -> ()
                n296 = local write "Move Up"(w690) -> ()
              }
            }
            n297 = call "Defer_FP_Updates.vi"("Defer Panel Updates"=FALSE, "error in"=w677, "lv_icon.vi in"=w683) -> ("error out"=w682:errorcluster)  [unwired: 8 out]
          }
          event User Event {
            # "This is an initialization event for the glyphs."
            n298 = event-data() -> ("Glyphs"=w705:string)  [unwired: 1 out]
            n299 = Unbundle By Name(w693) -> ("Ref.GlyphLoadAnimation"=w692:refnum<vi>, "Ref.refreshGlyphs"=w691:refnum<vi>)
            n300 = Unflatten From String(type=T34[] [], binary string=w705, error in (no error)=w703) -> (value=w700:T34[], error out=w702:errorcluster)  [unwired: 3 out]
            n301 = call "Populate Graphics.vi"("error in"=w702, "Glyphs []"=w700, "Data in"=w693) -> ("error out"=w701:errorcluster, "Data out"=w697:T28)  [unwired: 7 out]
            n302 = call "Write Glyphs to  File.vi"("File Name"="Glyphs.bin", "Path"=Pathes."Glyphs", "error in (no error)"=w701, "Graphics []"=w700) -> ("error out"=w696:errorcluster)  [unwired: 7 out]
            n303 = call "ChangeRefreshGraphicsState.vi"("error in (no error)"=w696, "refreshing?"=FALSE, "button ref"=w691, "animatedDecoration ref"=w692) -> ("error out"=w695:errorcluster)  [unwired: 7 in]
          }
          event "Glyphs": Mouse Down {
            n304 = event-data() -> ("CtlRef"=w707:refnum<vi>, "Coords"=w712:T31)  [unwired: 1 out]
            n305 = local write "Filter glyphs by keyword"("") -> ()
            n306 = call "Mouse Down_Tree.vi"("Tree"=w707, "error in (no error)"=w713, "Coords"=w712) -> ("error out"=w711:errorcluster)  [unwired: 8 out]
            n307 = call "Escape.vi"("error in"=w711, "Data in"=w709) -> ("error out"=w710:errorcluster, "Data out"=w708:T28)  [unwired: 1 in, 7 out]
          }
          event "Glyphs": Value Change {
            n308 = event-data() -> ("NewVal"=w721:string)  [unwired: 1 out]
            n309 = Unbundle By Name(w717) -> ("Class.Glyph"=w718:refnum<class "Glyph.lvclass">, "Ref.DNL_Glyphs []"=w714:refnum<vi>)
            n310 = call "FilterGlyphs.vi"("error in (no error)"=w719, "DNL_Glyphs []"=w714, "Tag"=w721, "Glyph in"=w718) -> ("error out"=w720:errorcluster, "Glyph out"=w716:refnum<class "Glyph.lvclass">)  [unwired: 6 out]
            n311 = Bundle By Name(cluster=w717, "Class.Glyph"=w716) -> (w715:T28)
          }
          event "Filter glyphs by keyword": Mouse Down {
            # "If a mouse down event should\nselect the entered text, enable this case"
            n312 = event-data() -> ("CtlRef"=w730:refnum<vi>)  [unwired: 1 out]
            n313 = disable-structure shown="Disabled" {
              disable-tunnel: w731 -> [w734 w737]
              disable-tunnel: w730 -> [w733 _]
              disable-tunnel: [w732 w737] -> w729
              frame Disabled {
                n314 = property class="Str"(reference=w733, error in=w734, "Text.Selection Start"=u32 0 ("Text.Selection:Start"), "Text.Selection End"=-1 ("Text.Selection:End")) -> (error out=w732:errorcluster)  [unwired: 1 out]
              }
              frame Enabled {
              }
            }
            n315 = call "Finalize Text.vi"("error in (no error)"=w729, "Data in"=w727) -> ("error out"=w728:errorcluster, "Data out"=w726:T28)  [unwired: 8 out]
            n316 = call "DeselectLayer.vi"("error in (no error)"=w728, "Data in"=w726) -> ("error out"=w725:errorcluster, "Data out"=w724:T28)  [unwired: 8 out]
            n317 = call "Escape.vi"("error in"=w725, "Data in"=w724) -> ("error out"=w722:errorcluster, "Data out"=w723:T28)  [unwired: 1 in, 7 out]
          }
          event "Filter glyphs by keyword": Value Change {
            n318 = event-data() -> ("NewVal"=w751:string)  [unwired: 1 out]
            n319 = Unbundle By Name(w746) -> ("Class.Glyph"=w747:refnum<class "Glyph.lvclass">, "Ref.DNL_Glyphs []"=w744:refnum<vi>, "Ref.Glyphs tree"=w743:refnum<vi>)
            n320 = First Call?() -> (First Call?: T/F=w749:bool)
            n321 = Not(x=w749) -> (.not. x?=w750:bool)
            n322 = call "SearchGlyphs.vi"("Glyphs tree"=w743, "DNL_Glyphs []"=w744, "Reset position? (F)"=w750, "error in (no error)"=w748, "Keyword"=w751, "Glyph in"=w747) -> ("error out"=w742:errorcluster, "Glyph out"=w745:refnum<class "Glyph.lvclass">)  [unwired: 4 out]
            n323 = Bundle By Name(cluster=w746, "Class.Glyph"=w745) -> (w739:T28)
            n324 = call "Set Undo Flag.vi"("error in"=w742, "Data in"=w739) -> ("error out"=w741:errorcluster, "Data out"=w740:T28)  [unwired: 8 in]
          }
          event "Glyphs []": Mouse Down {
            n325 = event-data() -> ("Button"=w760:u16, "Mods.Double Click"=w761:bool, "CtlRef"=w763:refnum<vi>, "Coords"=w764:T31)  [unwired: 1 out]
            n326 = case shown="1" w760 {
              tunnel: w764 -> [_ w773]
              tunnel: w763 -> [_ w772]
              tunnel: [w766 w771] -> w757
              tunnel: w762 -> [w766 w770]
              tunnel: w761 -> [_ w769]
              tunnel: w755 -> [w765 w768]
              tunnel: [w765 w767] -> w753
              frame 0, Default {
              }
              frame 1 {
                # "Left click"
                n327 = call "Mouse Down_Glyphs.vi"("Double Click"=w769, "Coords"=w773, "error in"=w770, "CtlRef"=w772, "Data in"=w768) -> ("error out"=w771:errorcluster, "Data out"=w767:T28)  [unwired: 1 in, 4 out]
              }
            }
            n328 = call "Reset layer template selection.vi"("error in (no error)"=w757, "Data in"=w753) -> ("error out"=w756:errorcluster, "Data out"=w754:T28)  [unwired: 1 in, 7 out]
            n329 = call "Update glyph path string.vi"("error in (no error)"=w756, "Data in"=w754) -> ("error out"=w758:errorcluster, "Data out"=w752:T28)  [unwired: 1 in, 7 out]
          }
          event Value Change {
            n330 = event-data() -> ()  [unwired: 2 out]
            n331 = Unbundle By Name(w776) -> ("Ref.GlyphLoadAnimation"=w774:refnum<vi>, "Ref.refreshGlyphs"=w775:refnum<vi>)
            n332 = call "Launch Dynamically Load Graphics.vi"("User events"=w777, "Path"=Pathes."Glyphs", "error in (no error)"=w779, "button ref"=w775, "animatedDecoration ref"=w774) -> ("error out"=w778:errorcluster)  [unwired: 1 in, 5 out]
          }
          event "Help": Value Change {
            n333 = event-data() -> ()  [unwired: 2 out]
            n334 = control-ref of="This VI"() -> (w783:refnum<vi>)
            n335 = property class="VI"(reference=w783) -> (error out=w781:errorcluster, "Help.URL"=w782:string)  [unwired: 1 in, 1 out]
            n336 = call "IE_Open Help Link.vi"("error in (no error)"=w781, "Help.URL"=w782) -> ()  [unwired: 9 in, 1 out]
          }
          event "Glyphs", "Templates": Item Close; "Glyphs", "Templates": event #0x1e {
            n337 = event-data() -> ("CtlRef"=w786:refnum<vi>)  [unwired: 1 out]
            n338 = call "DealWithScrollbars.vi"("error in (no error)"=w788, "Tree"=w786) -> ("error out"=w787:errorcluster)  [unwired: 9 in]
          }
        }
        n339 = case shown="False" w137 {
          tunnel: [_ w158] -> w139
          tunnel: w138 -> [w149 w155]
          tunnel: [w149 w160] -> w133
          tunnel: "Tools" -> [_ w159]
          tunnel: w147 -> [w148 w156]
          tunnel: [w148 w157] -> w146
          frame False {
          }
          frame True {
            n340 = call "Apply Body Text.vi"("error in"=w155, "Body Text"="Body Text", "Data in"=w156) -> ("error out"=w151:errorcluster, "Data out"=w153:T28)  [unwired: 2 in, 5 out]
            n341 = call "Add Data to History.vi"("error in"=w151, "Data in"=w153) -> ("error out"=w150:errorcluster, "Data out"=w152:T28)  [unwired: 8 in]
            n342 = call "DrawIcon.vi"("Tools"=w159, "error in (no error)"=w150, "Data in"=w152) -> ("error out"=w160:errorcluster, "Icon"=w158:picture, "Data out"=w157:T28, "RGB"=→"RGB":string, "XYL"=→"XYZ":string)  [unwired: 2 in, 2 out]
            "Icon" <- w158
            "Preview" <- w158
          }
        }
        n343 = Or(x=w133, y=w143) -> (x .or. y?=w142:bool)
      }
      n344 = call "Buffer for lossless tracking.vi"("Ref Cluster"=w118, "User events"=w106, "error in (no error)"=w122, "Buffer"=w121) -> ()  [unwired: 8 out]
      n345 = call "Extract LV Icon Data.vi"("error in (no error)"=w112, "LabVIEW Icon in (original)"=w110, "Data in"=w114) -> ("error out"=w111:errorcluster, "LabVIEW Icon out"=w113:string, "Data out"=w109:T28)  [unwired: 6 in]
      n346 = call "Get Image Data.vi"("Pic In"=w105) -> ("image data out"=w117:T2)  [unwired: 2 in, 8 out]
      n347 = call "Get Image Data.vi"("depth (24)"=1 ("depth"), "Pic In"=w105) -> ("image data out"=w127:T2)  [unwired: 2 in, 7 out]
      n348 = call "SetCursor.vi"("Radio Buttons"=Tools."Select", "Data in"=w109) -> ("Data out"=w108:T28)  [unwired: 8 in, 1 out]
      n349 = Unbundle By Name(w111) -> ("code"=w129:i32)
      n350 = flat-sequence {
        tunnel: w132 -> [w791]
        tunnel: w130 -> [w799]
        tunnel: w111 -> [w798]
        tunnel: w106 -> [w796]
        tunnel: w108 -> [w792]
        frame #0 {
          # "Make sure the Keep IE in Memory VI runs and completes before the main Icon Editor panel is closed."
          n351 = Unbundle By Name(w796) -> ("Global stop?"=w795:refnum<user-event>, "Templates"=w794:refnum<user-event>, "Glyphs"=w793:refnum<user-event>)
          n352 = call "Write INI Tokens and VI Tags.vi"("error in"=w798, "Global Data in"=w792) -> ()  [unwired: 1 in, 9 out]
          n353 = Unregister For Events(event registration refnum=w791) -> ()  [unwired: 1 in, 1 out]
          n354 = Release Notifier(notifier=w799, force destroy? (F)=TRUE) -> ()  [unwired: 1 in, 3 out]
          n355 = global read "Data.vi" "Debug"() -> (w790:bool)
          n356 = Generate User Event(user event=w795, event data cluster=TRUE) -> ()  [unwired: 2 in, 2 out]
          n357 = Destroy User Event(user event=w794) -> ()  [unwired: 1 in, 1 out]
          n358 = Destroy User Event(user event=w793) -> ()  [unwired: 1 in, 1 out]
          n359 = case shown="False" w790 {
            frame False {
              n360 = call "Call Keep IE in Memory.vi"() -> ()  [unwired: 1 out]
            }
            frame True {
            }
          }
        }
        frame #1 {
          n361 = global read "Data.vi" "Debug"() -> (w801:bool)
          n362 = case shown="False" w801 {
            frame False {
              n363 = invoke class="VI" method="FP.Close"() -> ()  [unwired: 3 in, 3 out]
            }
            frame True {
            }
          }
        }
      }
      n364 = call-dynamic "GET_Notifier.vi"("error in (no error)"=w115, "Ants.lvclass in"=w119) -> ("error out"=w125:errorcluster, "Notifier"=w130:refnum<notifier>, "Ants.lvclass out"=w126:refnum<class "Ants.lvclass">)  [unwired: 7 out]
      n365 = call "RunningAnts.vi"("error in (no error)"=w125, "Ants in"=w126) -> ()  [unwired: 10 out]
    }
    frame Error {
      n366 = Unbundle By Name(w803) -> ("code"=w804:i32)
      n367 = call <vilib>:"Simple Error Handler.vi"("error in (no error)"=w803) -> ()  [unwired: 4 in, 5 out]
    }
  }
  "BW icon out" <- w69
  "Error code out" <- w73
  "Color icon out" <- w51
  "LabVIEW Icon out" <- w48
